vi "WHD_VEten_0.1.6.WS_BIDIR_Cal_26_01_2024.vi"() -> ()   [LabVIEW 2015]
uses:
  <vilib>/LabVIEW Targets/FPGA/cRIO/shared/nicrio_ModuleControls/nicrio_cRIO-9234_DataRatesRing2.ctl
  <vilib>/RTwatchdog.llb/Watchdog expiration actions.ctl
  <vilib>/userdefined/High Color/nirio_resource_hc.ctl
  <vilib>/Platform/TimedLoop/XDataNode/timing_clust.ctl
  <vilib>/Platform/TimedLoop/XDataNode/nitl_modes.ctl
  <vilib>/Platform/TimedLoop/XDataNode/wakeup.ctl
  <vilib>/Analysis/5stat.llb/RMS (DBL).vi
  <vilib>/FPGAPlugInAG/cRIO-9031/niLvFpga_Open_cRIO-9031.vi
  <vilib>/Utility/error.llb/Error Cluster From Error Code.vi
  <vilib>/rvi/errors/niLvFpgaAdjustHostInterfaceError.vi
  <vilib>/FPGAPlugInAG/cRIO-9031/niLvFpga_Run_cRIO-9031.vi
  <vilib>/rvi/interface/common/niFpgaWaitOnOcc.vi
  <vilib>/Utility/file.llb/Write Delimited Spreadsheet (string).vi
  <vilib>/FPGAPlugInAG/cRIO-9031/niLvFpga_Reset_cRIO-9031.vi
  <vilib>/measure/madcrms.llb/Basic Averaged DC-RMS for 1 Chan.vi
  <vilib>/measure/maspectr.llb/FFT Spectrum (Mag-Phase) for 1 Chan.vi
  <vilib>/Utility/config.llb/Write Key (Double).vi
  <vilib>/FPGAPlugInAG/cRIO-9031/niLvFpga_Close_cRIO-9031.vi
  <vilib>/rvi/interface/nirviOpenFPGA/nirviOpenFPGA.xnode
  FPGA Bitfiles/WRDArabia_FPGATarget_FPGA8a2wsBIdirec_pdg683fU6LY.lvbitx
  <vilib>/rvi/interface/nirviReadWriteControl/nirviReadWriteControl.xnode
  <vilib>/rvi/interface/nirviMethod/nirviMethod.xnode
  <vilib>/platform/TimedLoop/XDataNode/XDataNode.xnode
  <vilib>/rvi/interface/nirviCloseFPGA/nirviCloseFPGA.xnode
  <vilib>/NI_Real-Time Target Support.lvlib
  <vilib>/rvi/errors/niLvFpgaMergeErrorWithErrorCode.vi
  AURA_Wheel/Json2Labv.lvlib
  AURA_Wheel/AuraWheelAPI/AuraWheel.lvlib
  NiFpgaLv.dll
  <vilib>/FPGAPlugInAG/cRIO-9031/niLvFpga_ConfigureFifo_cRIO-9031.vi
  <vilib>/FPGAPlugInAG/cRIO-9031/niLvFpga_StartFifo_cRIO-9031.vi
  <vilib>/FPGAPlugInAG/cRIO-9031/niLvFpga_ReadFifo_cRIO-9031.vi
  <vilib>/FPGAPlugInAG/cRIO-9031/niLvFpga_StopFifo_cRIO-9031.vi
  <vilib>/measure/NI_MAPro.lvlib
  <vilib>/Analysis/NI_AALPro.lvlib
  <vilib>/Analysis/NI_AALBase.lvlib
  <vilib>/Utility/config.llb/NI_LVConfig.lvlib
  <vilib>/Platform/TimedLoop/XDataNode/XDNodeRunTimeDep.lvlib
  Library/IF2_Reader/IF2_Reader.lvlib
panel:
  out "t":string
  out "Diagnostic data":sgl[](array[numeric])
  out "Last Train passes - RFIDs":T1
  out "I2":sgl[](array[numeric])
  out "I1":sgl[](array[numeric])
  out "A8":sgl[](array[numeric])
  out "A7":sgl[](array[numeric])
  out "A6":sgl[](array[numeric])
  out "A5":sgl[](array[numeric])
  out "A4":sgl[](array[numeric])
  out "A3":sgl[](array[numeric])
  out "A2":sgl[](array[numeric])
  out "A1":sgl[](array[numeric])
  out "Accelerometer 8":bool
  out "Accelerometer 7":bool
  out "Accelerometer 6":bool
  out "Accelerometer 5":bool
  out "Accelerometer 4":bool
  out "Accelerometer 3":bool
  out "Accelerometer 2":bool
  out "Accelerometer 1":bool
  out "Wheel detector 2":bool
  out "Wheel Detector 1":bool
  out "Last time checked":string
  out "RFID connection":bool
  out "Internet connection":bool
  out "Inicio diagnosis":timestamp
  out "RFID_status":path=path "c:/RFID/status.csv"
  in  "Diagnosis":bool
  out "T fuera rango":bool
  out "Frequency":dbl[](array[numeric])
  out "Value to compare":dbl[](array[numeric])
  in  "Developer password":string
  out "Waveform Graph":waveform(sgl)[](graph)
  out "min":dbl[](array[numeric])
  out "max":dbl[](array[numeric])
  out "median":dbl[](array[numeric])
  out "mean":dbl[](array[numeric])
  in  "Accelerometer":i32=1 min=1 max=8
  out "Low cutoff freq":dbl
  out "noise_range":dbl
  out "Numeric":i32
  out "Calibration parameter":dbl
  out "Accel.detected":i32
  out "Mean\nfrequency":dbl format="%0.2f"
  out "Nº meas":i32
  out "Array":i32[](array[numeric])
  out "sorted array":i32[](array[numeric])
  out "Array 3":i32[](array[numeric])
  out "max value":i32
  out "max index(es)":i32
  out "element":i32
  out "size(s) 3":i32
  out "size(s)":i32[](array[numeric])
  out "Valid\nindex":i32[](array[numeric])
  out "Acquiring time":dbl
  out "Inicio pasada 2":timestamp
  out "calibration log":path
  out "date/time string 2":string
  out "Folder":path
  in  "Developer commad":string
  out "Save calibration":bool
  out "Pattern amplitude (g)":dbl=1.02
  out "Pattern frequency (Hz)":dbl=159.2
  out "Report":string
  out "AURA wheel test":bool
  out "LOG.txt":path
  out "Report_AURA":string
  out "error FPGA":errorcluster
  out "error AURA":errorcluster
  out "error manipulacion archivos":errorcluster
  out "Response headers":string
  out "Max RMS Ruedas":dbl[][](array[numeric])
  out "TAGs LR6":string[](array[string])
  out "TAGs HEX":string[](array[string])
  out "Parar":bool
  out "result":bool
  out "TAGs":string[](array[string])
  out "Temperatura (ºC)":dbl
  out "V (m/s)":dbl
  out "Digital?":bool=TRUE
  out "Watchdog config":T2={"reset"=FALSE, "occurrence"=FALSE, "trigger protocol"=enum."active high", "trigger line"=enum."none", "disable watchdog on VI exit"=TRUE}
  out "Tiempo de adquisicion":dbl=10.0
  out "Adquirir":bool
  out "Nº Ruedas 1":i32
  out "NºRuedas 2":i32
  out "Disco Duro Disponible (bytes)":i64
  out "Buffer Overflow":bool
  out "Buffer Underflow":bool
  out "Archivo\nvalido?":bool
  out "Número de ejes detectados":i32
  out "Ejes_convoy":i32
  out "Tiempo de paso (s)":dbl
  out "created path":path
  out "Nombre de archivo":path[](array[path])
  out "LR6 IP address":string="192.168.106.94"
  out "Port LR6":u16=2001
  out "Frecuencia de muestreo (Hz)":dbl=25600.0
  out "Escaneos de la FIFO por canal":u32=5000
  out "Tiempo extra al detector de paso (s)":dbl=1.0
  out "dt RMS":dbl=256.0
  out "Frecuencia de muestreo y módulo CRIO":T3=2 items=["51.200 kS/s (NI 9234)"=1, "25.600 kS/s (NI 9234)"=2, "17.067 kS/s (NI 9234)"=3, "12.800 kS/s (NI 9234)"=4, "10.240 kS/s (NI 9234)"=5, "8.533 kS/s (NI 9234)"=6, "7.314 kS/s (NI 9234)"=7, "6.400 kS/s (NI 9234)"=8, "5.689 kS/s (NI 9234)"=9, "5.120 kS/s (NI 9234)"=10, "4.654 kS/s (NI 9234)"=11, "4.267 kS/s (NI 9234)"=12, "3.938 kS/s (NI 9234)"=13, "3.657 kS/s (NI 9234)"=14, "3.413 kS/s (NI 9234)"=15, "3.200 kS/s (NI 9234)"=16, "3.012 kS/s (NI 9234)"=17, "2.845 kS/s (NI 9234)"=18, "2.695 kS/s (NI 9234)"=19, "2.560 kS/s (NI 9234)"=20, "2.438 kS/s (NI 9234)"=21, "2.328 kS/s (NI 9234)"=22, "2.226 kS/s (NI 9234)"=23, "2.133 kS/s (NI 9234)"=24, "2.048 kS/s (NI 9234)"=25, "1.969 kS/s (NI 9234)"=26, "1.896 kS/s (NI 9234)"=27, "1.829 kS/s (NI 9234)"=28, "1.765 kS/s (NI 9234)"=29, "1.707 kS/s (NI 9234)"=30, "1.652 kS/s (NI 9234)"=31]
  out "Puerto RFID":u16=2189
  out "IP RFID":string="192.168.106.99"
  out "Offset_rueda WS 2":fxp<+/-,24,-4>=0.004999998956918716 format="%.27g"
  out "Count(mSec)":u32=2
  out "RFID NEM on?":bool
  out "RFID LR6 on?":bool
  out "Canal cero WS1?":bool
  out "Canal cero WS2":bool
  in  "Calibration":bool
  out "Direccion 0?":bool
  out "Boton Adquirir?":bool
  out "RuedaDetectada2?":bool=TRUE
  out "RuedaDetectada1?":bool=TRUE
  out "Timeout ruedas":dbl
  out "Borrar archivos\nadquisicion con error":bool
  out "Able watchdog?":bool
  out "Reset watchdog?":bool
  out "Leer config RFID NEM":bool
  out "bytes to read":i32
  out "DeviceAddress":u8
  out "timeout ms (60000)":i32
  out "Max archivos":u32=2
  out "Bytes libre despues de borrar":u32=2
  out "Bytes min libre":u32=2
  out "Nº de acelerómetros":i32
  out "Nº inductivos":i32
  out "Offset_rueda WS 1":fxp<+/-,24,-4>=0.004999998956918716 format="%.27g"
  out "TAGs_AURAwheel":string[][](array[string])
  out "Plataformas?":bool
  out "Nº Ejes":i32[](array[numeric])
  out "Nº UTs":i32
  out "it-read-LR6":i32[](array[numeric])
  out "it-LR6":i32
  out "RFID_LR6_Error":errorcluster
  out "Series_flota":string[](array[string])
  out "Tabla_flota":string[][](array[string])
  out "Puntos medios de las ventanas":dbl[][](array[numeric])
  out "configuration file path":path=path "c:/Parametros.cfg"
  out "IP synchr":string
  out "data":cluster{"status":string}
  out "confRFID":path=path "c:/RFID/TAGS.csv"
  out "TAGS leidos":path=path "c:/RFID/TAGS.csv"
  out "Use Aura?":bool
  out "Parametros AuraWheel":string[](array[string])
  out "Parámetros acelerómetros":dbl[](array[numeric])
  out "Fin":bool
  out "Contador":i32=1
  out "Path LOG":path=path "c:/TEST"
  out "Fallo fotocelula":bool
  out "Path_Borrar":path=path "c:/Trenes"
  out "Longitud de la unidad":dbl
  out "Aviso no detección":string
  out "Time to Acquire Block (ms)":i32
  out "Distancia de acelerómetros":dbl[](array[numeric])
  out "Block Size":u32
  out "Distancias generales":dbl[](array[numeric])
  out "Reset del controlador":bool
  out "Parar la aplicación":bool
  out "date/time string":string
  out "Timeout ruedas":bool
  out "Tiempo":dbl
  out "Inicio pasada":timestamp
  out "Ultimo TEST":timestamp
  out "Fuente":bool=TRUE
  out "DC OK":string
  out "Aviso temperatura":string
  out "connection ID":refnum<k5>
  # "To check the status of the UPS please check the following LEDs physically in the system:"
  # "10. Bar graph showing the current available supply of the UPS (each bar is a 20%)"
  # "12. Red LED: alarm"
  # "13. Yellow LED: battery working mode"
  # "16. Green LED: Power In OK, mains mode"
  # "Calibration - Noise analysis"
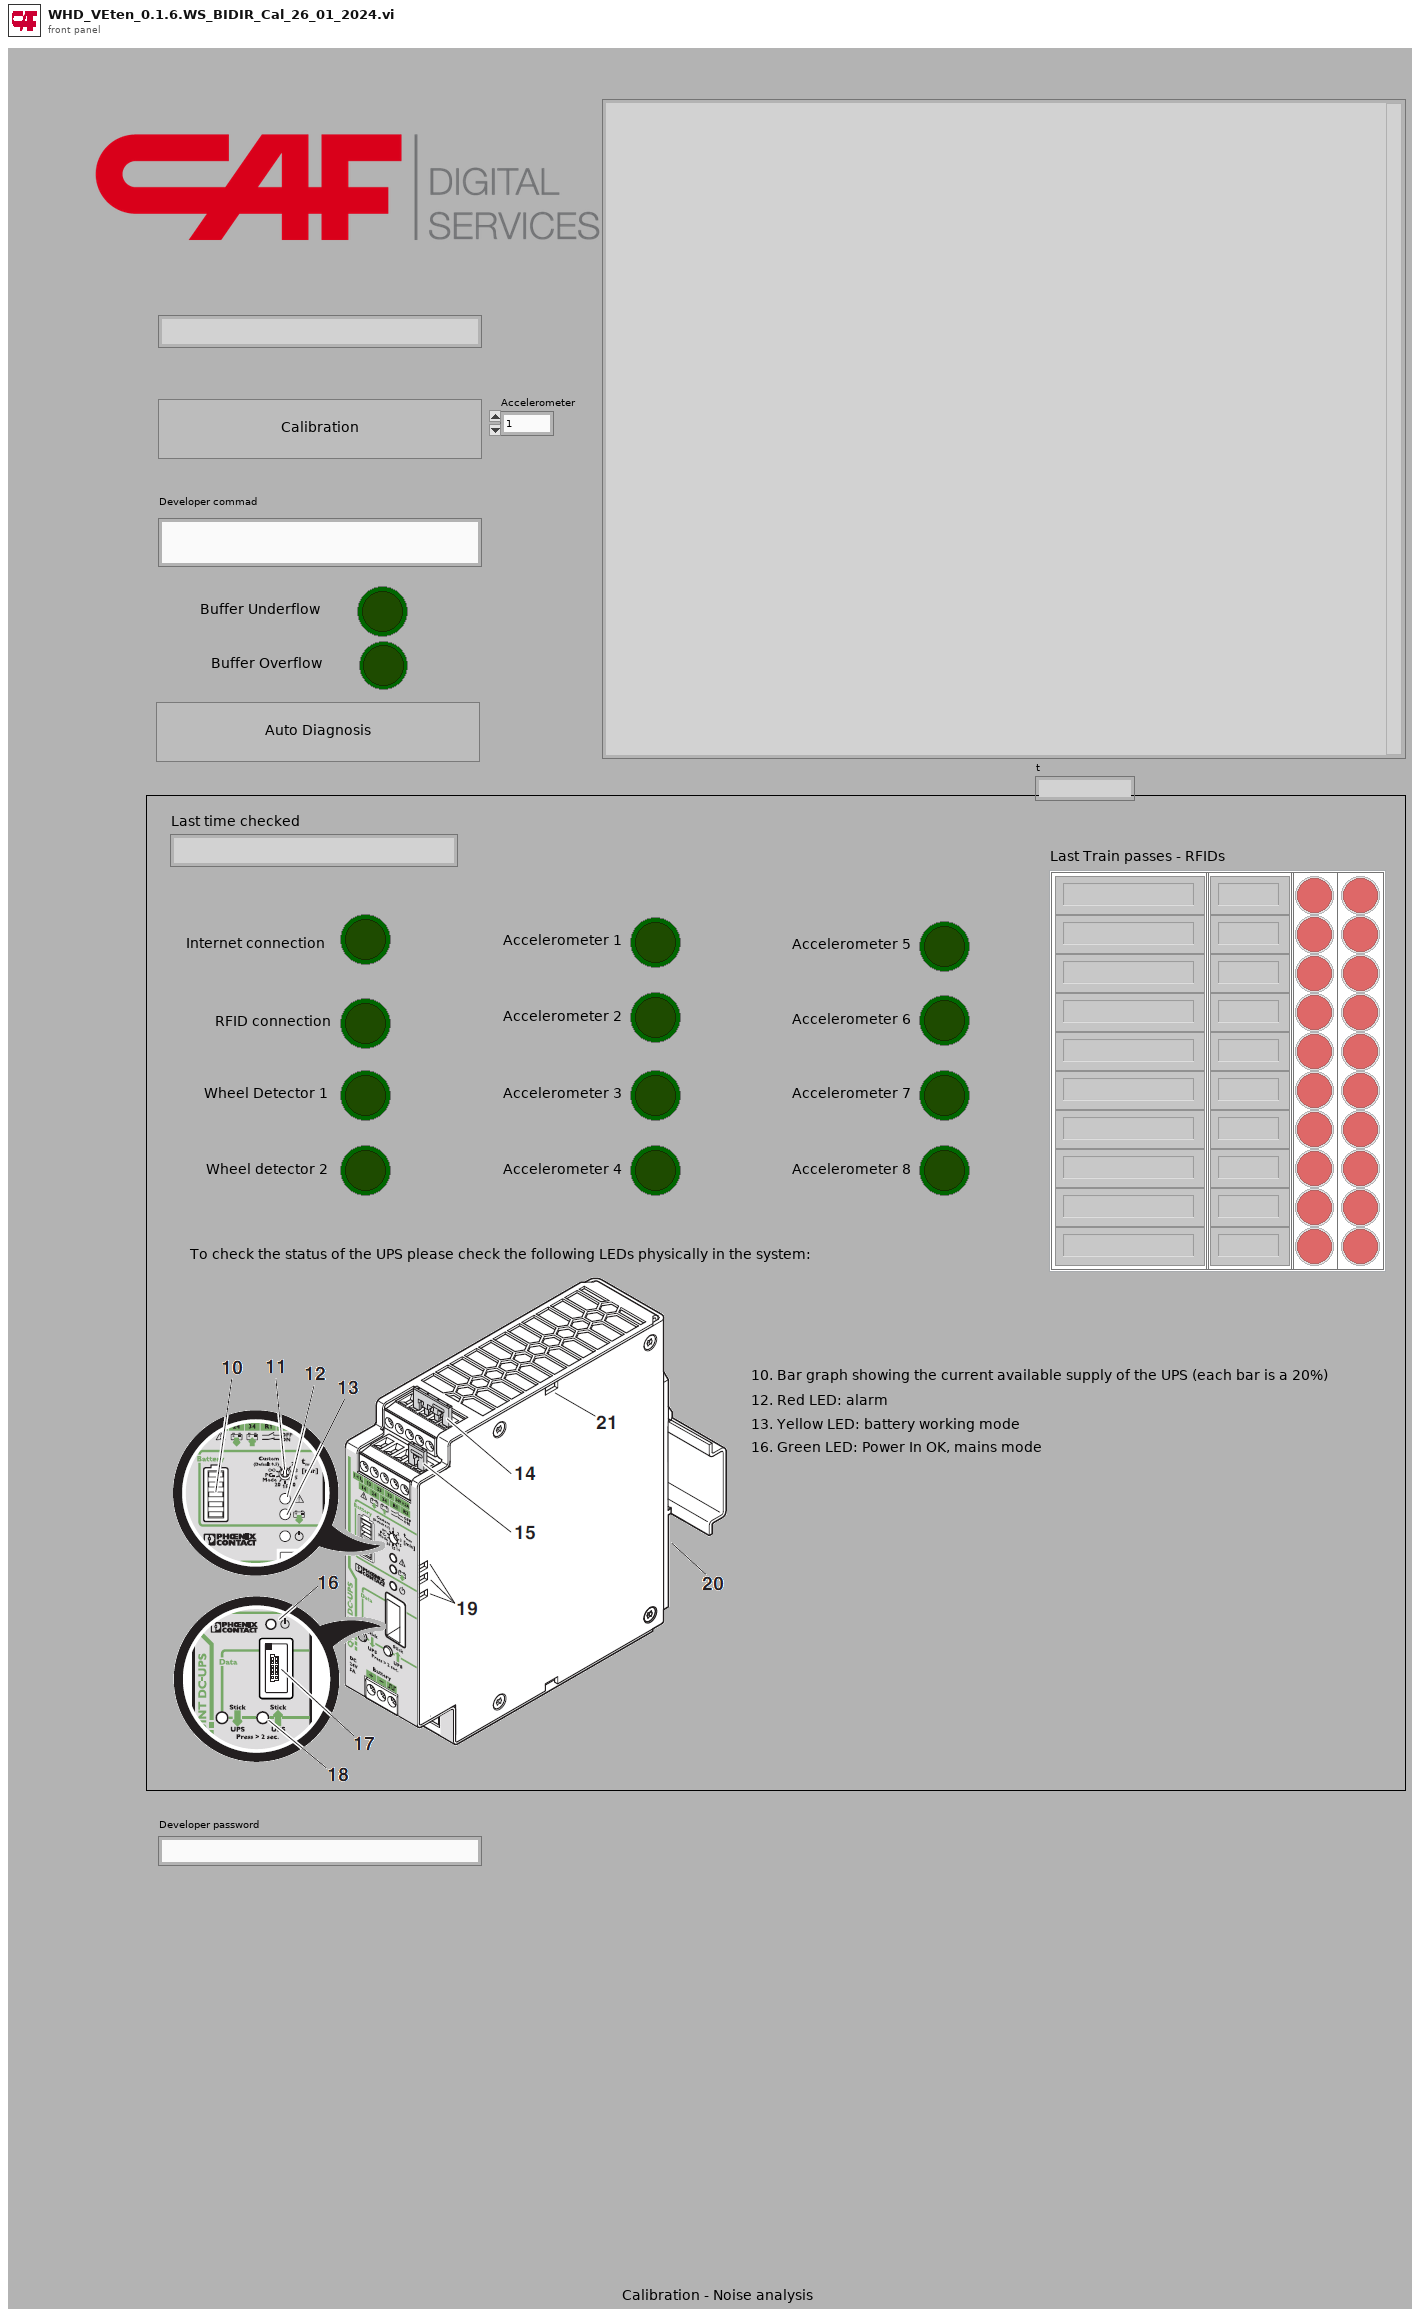
[diagram p1: front panel]
types:
  T1 = cluster{"Array 3":bool[], "Array 4":string[], "Array 6":string[], "Array 5":bool[]}
  T2 = typedef "Watchdog expiration actions.ctl" = cluster{"reset":bool, "occurrence":bool, "trigger protocol":enum16{"active high", "active low", "open collector"}, "trigger line":enum16{"none", "line 0", "line 1", "line 2", "line 3", "line 4", "line 5", "line 6", "line 7", "SMB line 0"}, "disable watchdog on VI exit":bool}
  T3 = typedef "nicrio_cRIO-9234_DataRatesRing2.ctl" = u8
  T4 = typedef "nirio_resource_hc.ctl" = tag
  T5 = enum16{"open", "replace", "create", "open or create", "replace or create", "replace or create with confirmation"}
  T6 = enum16{"big-endian, network order", "native, host order", "little-endian"}
  T7 = typedef "XDNodeRunTimeDep.lvlib/timing_clust.ctl" = cluster{"Expected End [f-1]":u64, "Actual End [f-1]":u64, "Finished Late? [f-1]":bool, "Expected End [i-1]":u64, "Actual End [i-1]":u64, "Finished Late? [i-1]":bool, "Expected Start [i]":u64, "Actual Start [i]":u64, "Expected Start [f]":u64, "Actual Start [f]":u64, "Source Name":string, "Structure Name":string, "Period":i64, "Deadline":i64, "Offset":i64, "Start":i64, "Priority":i32, "Timeout":i32, "Mode":T8, "Wakeup Reason":T9, "Error":errorcluster, "Source Type":string, "Secondary Source Type":string, "Global End Time":u64, "Global Start Time":u64, "Frame Duration":u64, "Iteration Duration":u64, "Assigned CPU":i32, "I/O Scan Engine Mode":u32}
  T8 = typedef "XDNodeRunTimeDep.lvlib/nitl_modes.ctl" = enum32{"No Change", "Process missed periods, maintain original phase", "Discard missed periods, maintain original phase", "Process missed periods, ignore original phase", "Discard missed periods, ignore original phase"}
  T9 = typedef "XDNodeRunTimeDep.lvlib/wakeup.ctl" = enum32{"Normal", "Aborted", "Asynchronous wakeup", "Timing source error", "Timed loop error", "Timeout"}
  T10 = cluster{"error IO":errorcluster, bool[], u32[], string[], dbl[]}
  T11 = cluster{"error out":errorcluster, dbl[], "Normalized Tags":string[], "Direccion 0?":bool}
  T12 = cluster{"g_ts":dbl, "p_sp":dbl, "p_tp":dbl, "p_tg":cluster{"tg_n":dbl, "tg_t":string}[], "p_ax":cluster{"ax_n":dbl, "ax_sp":dbl, "ax_wh":cluster{"wh_p":dbl, "wh_a1":dbl, "wh_a2":dbl, "wh_a3":dbl, "wh_a4":dbl}[]}[]}
  T13 = typedef "NI_LVConfig.lvlib/Config Data RefNum.ctl" = refnum<k1>
  T14 = cluster{"IP":string, "Port":u16, "ReaderConfigFile":path, "ROspecConfigFile":path}
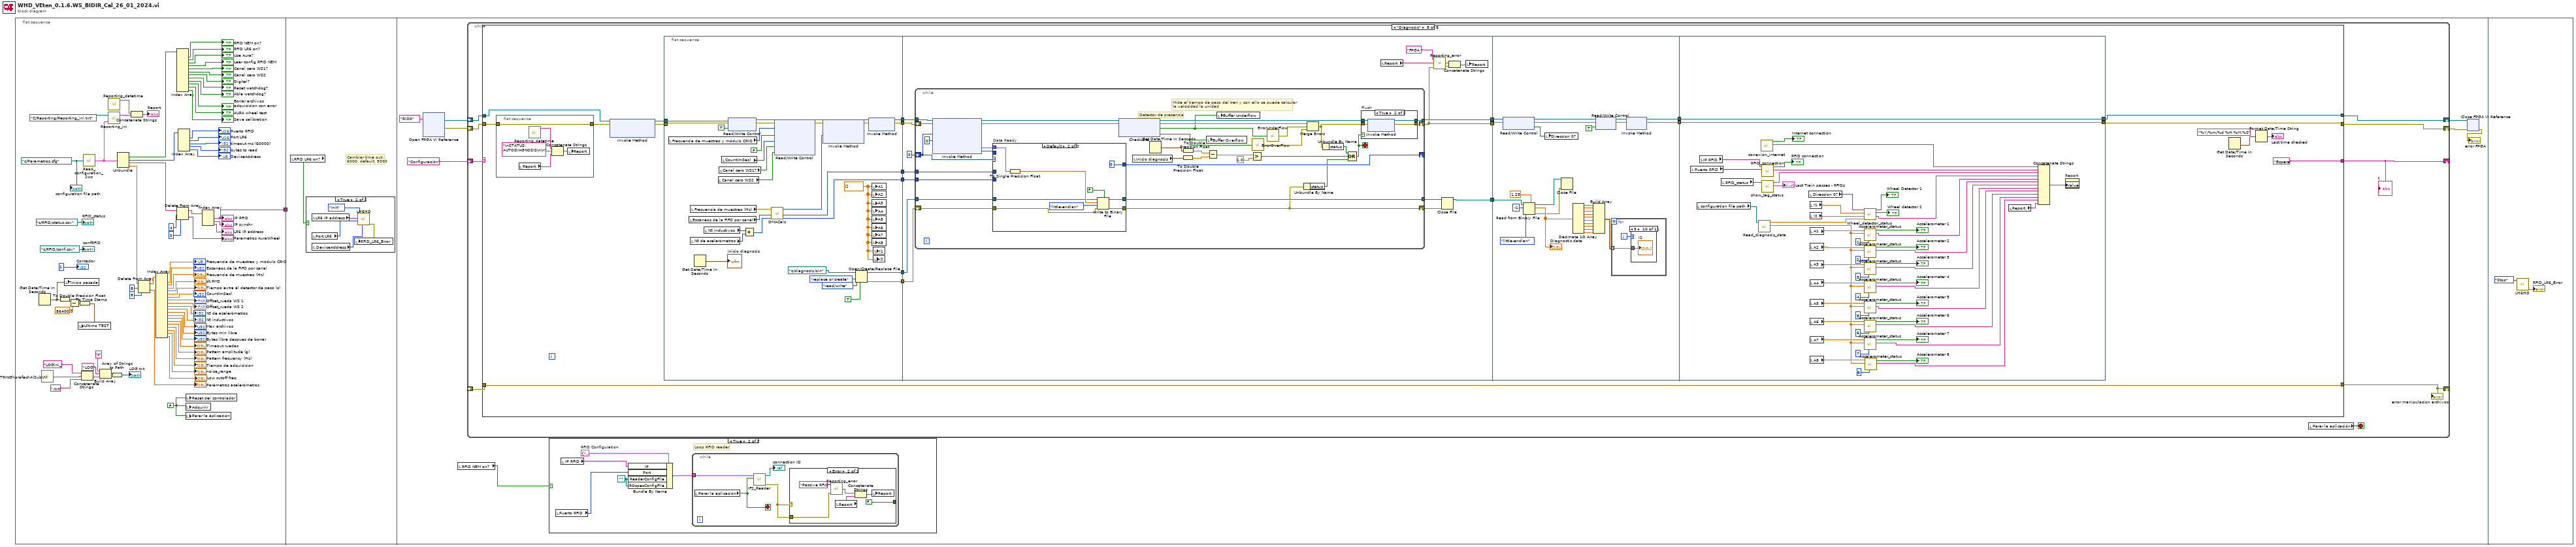
[diagram p0: block diagram]
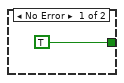
[diagram p4: hidden frame]
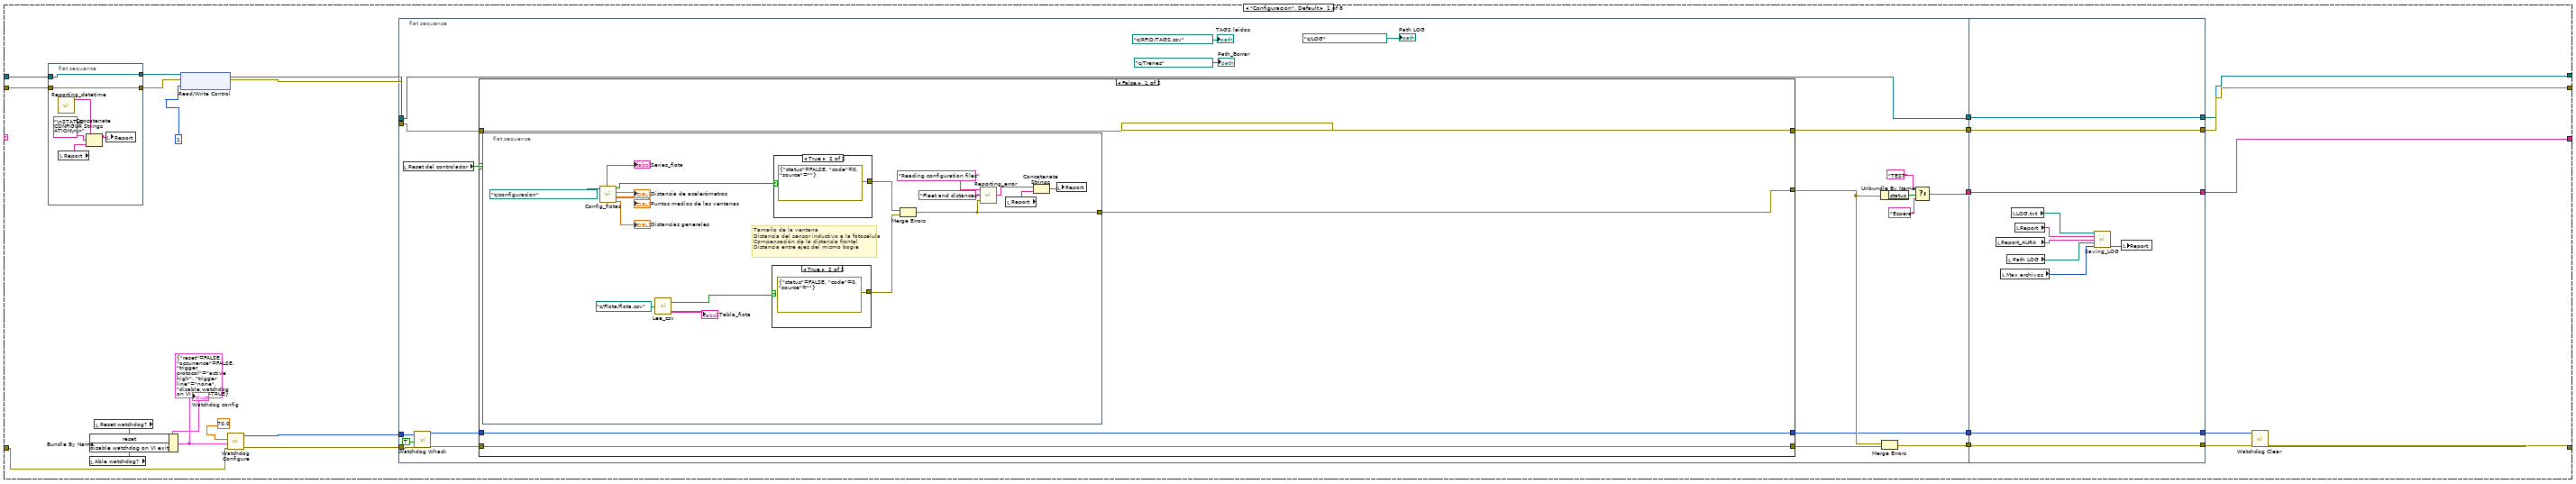
[diagram p5: hidden frame]
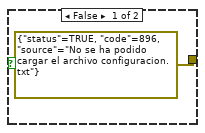
[diagram p6: hidden frame]
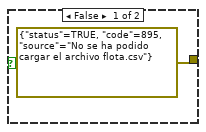
[diagram p7: hidden frame]
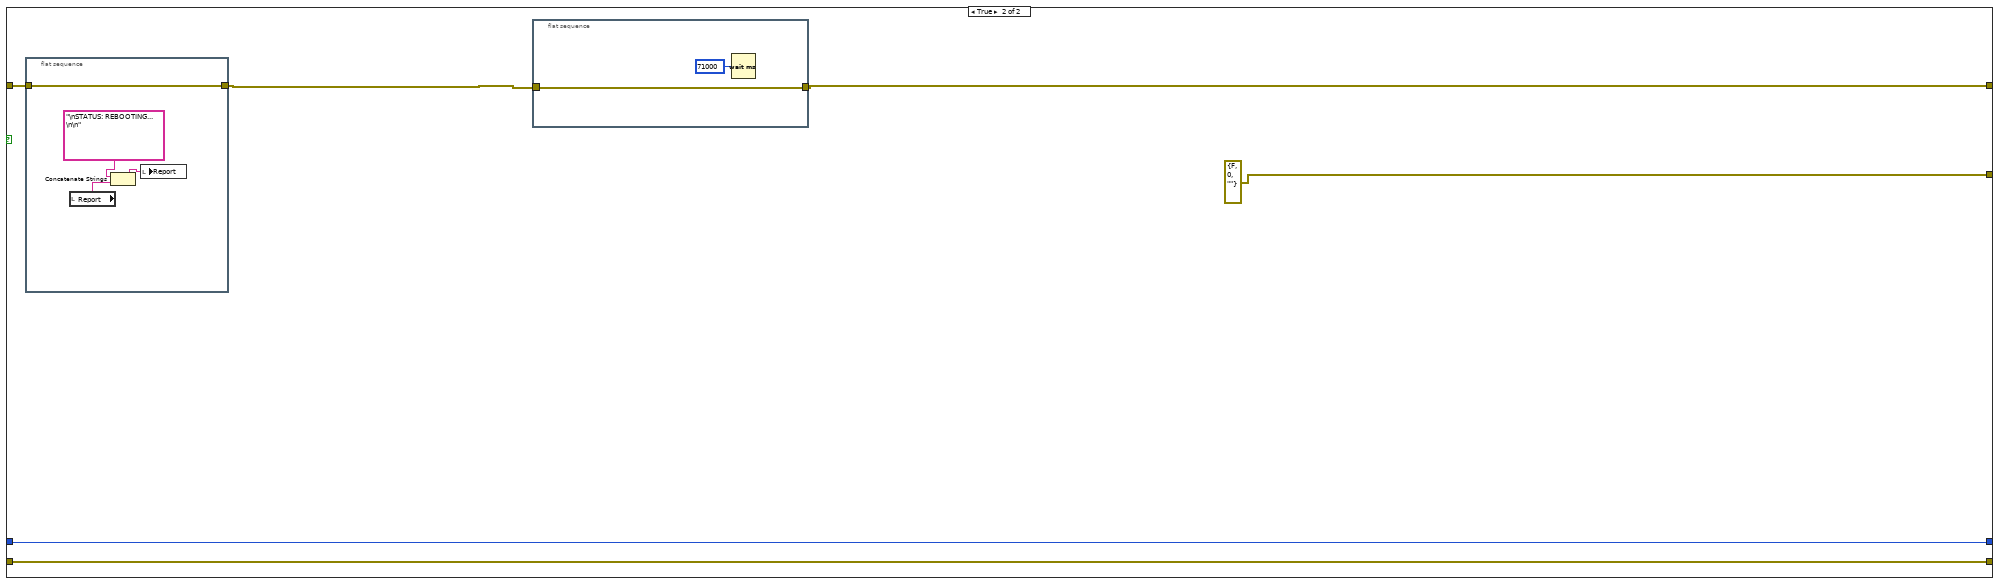
[diagram p8: hidden frame]
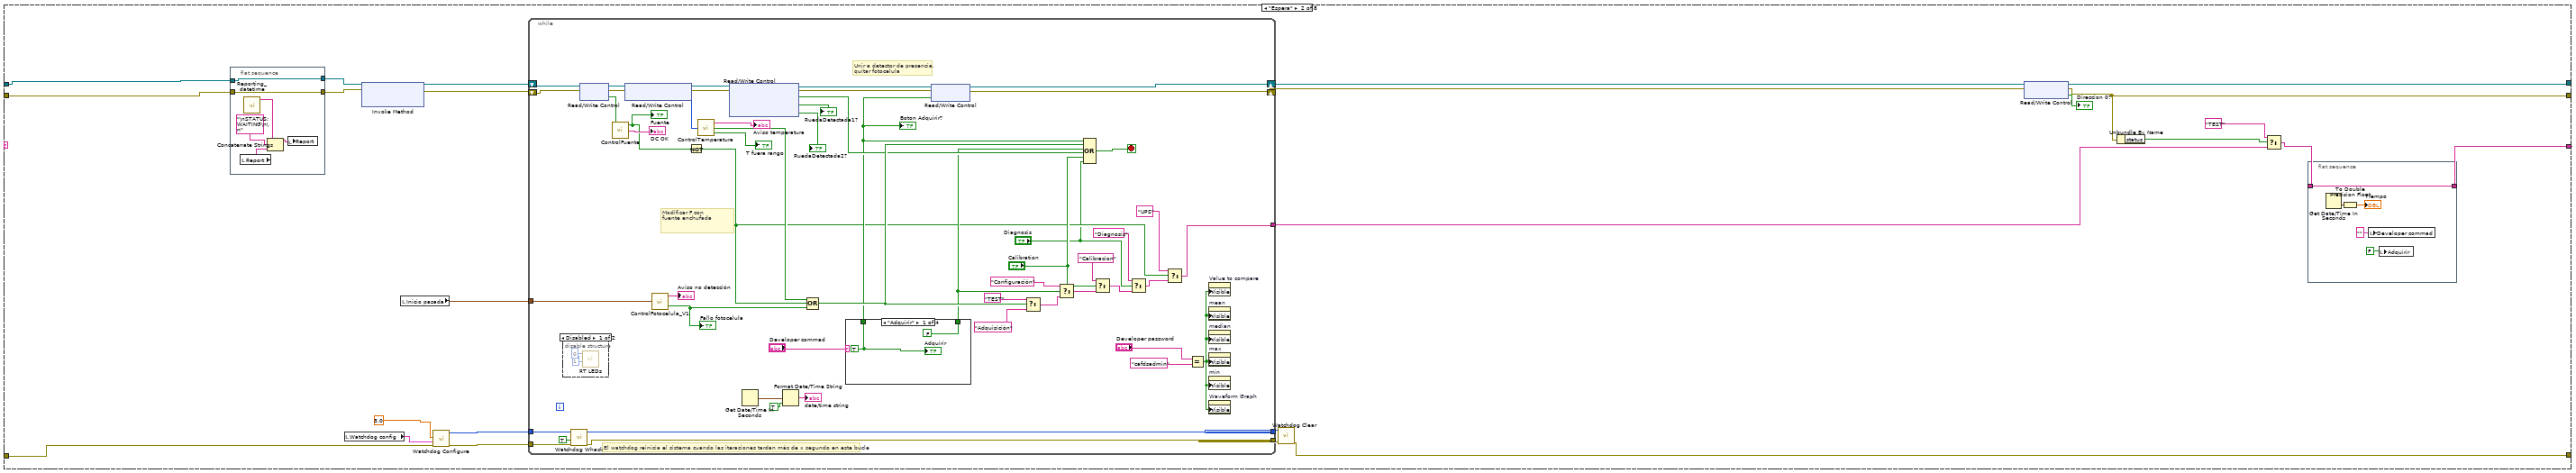
[diagram p9: hidden frame]
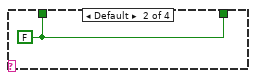
[diagram p10: hidden frame]
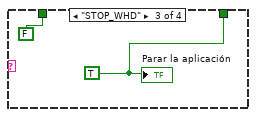
[diagram p11: hidden frame]
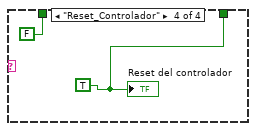
[diagram p12: hidden frame]
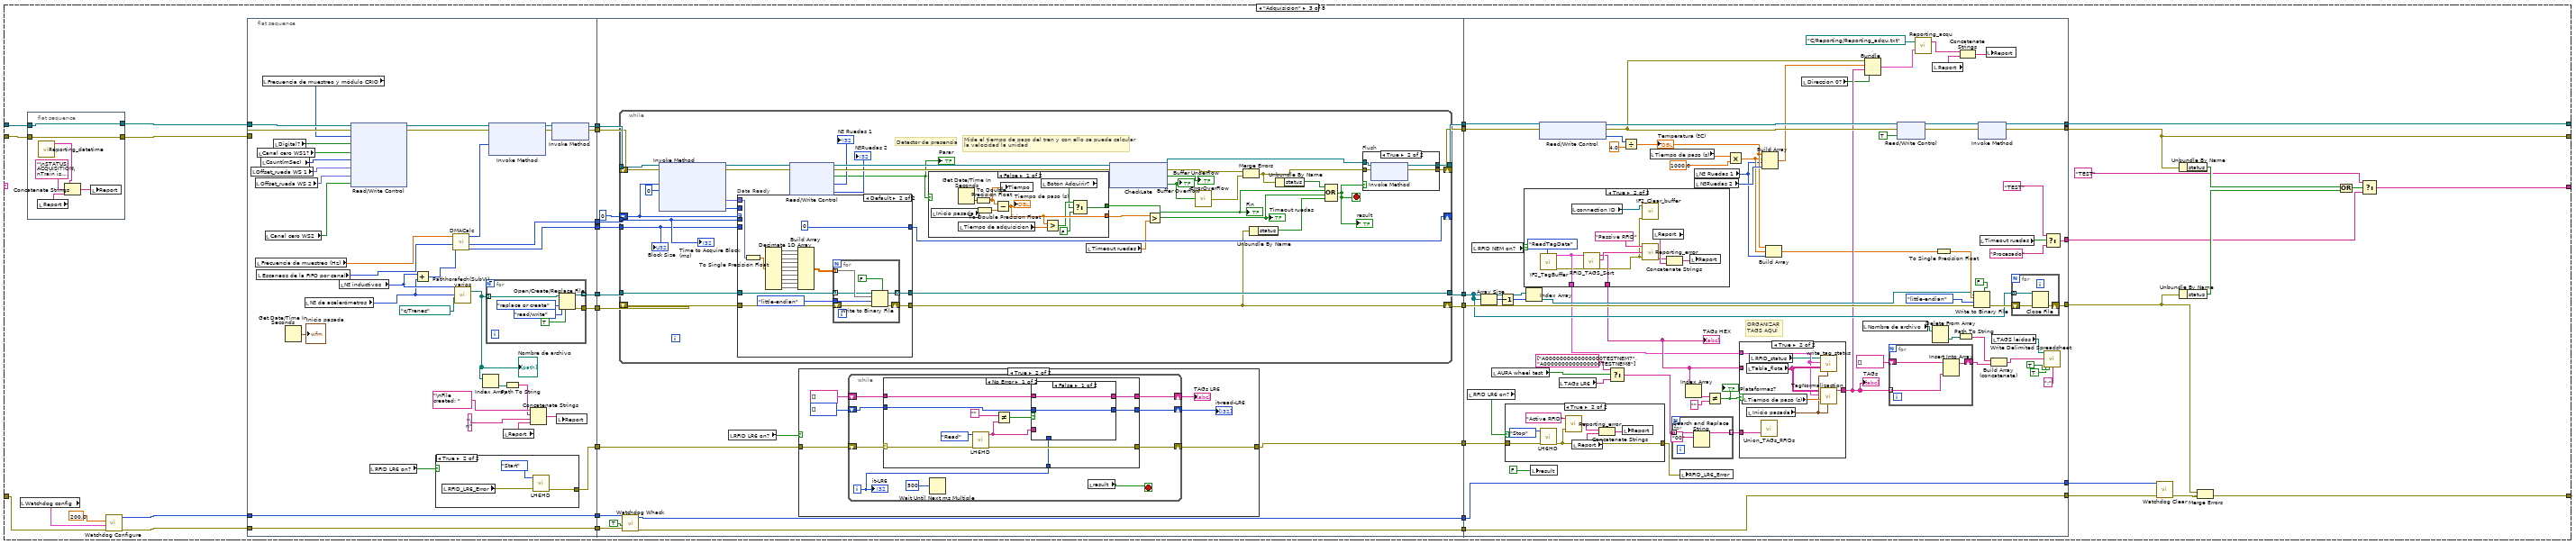
[diagram p14: hidden frame]
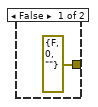
[diagram p15: hidden frame]
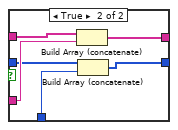
[diagram p17: hidden frame]
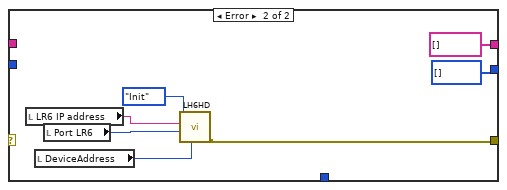
[diagram p18: hidden frame]
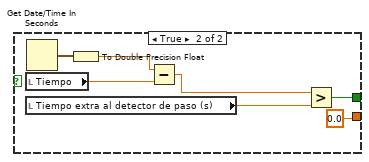
[diagram p19: hidden frame]
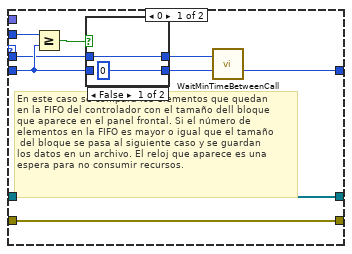
[diagram p20: hidden frame]
diagram:
  n1 = flat-sequence {
    tunnel: [w5] -> w1
    tunnel: w1 -> [_]
    frame #0 {
      w6 = FALSE ("Reset del controlador")
      w67 = path "c:/Parametros.cfg" ("configuration file path")
      n2 = Get Date/Time In Seconds() -> (seconds since 1Jan1904=w72:timestamp)
      n3 = call "STRINGhorafechA(SubVI).vi"() -> ("STRINGhora_fecha"=w17:string)
      n4 = To Double Precision Float(number=w72) -> (double precision float=w74:dbl)
      n5 = local write "Inicio pasada"(w72) -> ()
      n6 = Subtract(x=w74, y=86400.0) -> (x-y=w73:dbl)
      n7 = To Time Stamp(1:w73) -> (0:w71:timestamp)
      n8 = local write "Ultimo TEST"(w71) -> ()
      n9 = Concatenate Strings("LOGini_" ("string"), w17, ".txt" ("string")) -> (w19:string)
      n10 = call "Read_configuration_2ws.vi"("configuration file path"=w67) -> ("output cluster"=w23:T10)
      n11 = Build Array("c", "LOG" ("element"), w19) -> (w16:string[])
      n12 = call "Reporting_ini.vi"("Configuration cluster"=w23, "address repoting"=path "C:/Reporting/Reporting_ini.txt" ("file (use dialog)")) -> ("Reporting"=w22:string)  [unwired: 1 in]
      n13 = call "Reporting_datetime.vi"() -> ("String"=w20:string)  [unwired: 11 in]
      n14 = Array of Strings to Path(0:w16) -> (2:→"LOG.txt":path)  [unwired: 1 out]
      n15 = Unbundle(w23) -> (w70:bool[], w69:u32[], w62:string[], w66:dbl[])  [unwired: 1 out]
      n16 = Concatenate Strings(w20, w22) -> (→"Report":string)
      n17 = Delete From Array(array=w66, length=8, index=8) -> (deleted portion=→"Parámetros acelerómetros":dbl[], array with subset deleted=w65:dbl[])
      n18 = Index Array(array=w65) -> (element #1=→"Frecuencia de muestreo y módulo CRIO":dbl, element #2=→"Escaneos de la FIFO por canal":dbl, element #3=→"Frecuencia de muestreo (Hz)":dbl, element #4=→"dt RMS":dbl, element #5=→"Tiempo extra al detector de paso (s)":dbl, element #6=→"Count(mSec)":dbl, element #7=→"Offset_rueda WS 1":dbl, element #8=→"Offset_rueda WS 2":dbl, element #9=→"Nº de acelerómetros":dbl, element #10=→"Nº inductivos":dbl, element #11=→"Max archivos":dbl, element #12=→"Bytes min libre":dbl, element #13=→"Bytes libre despues de borrar":dbl, element #14=→"Timeout ruedas":dbl, element #15=→"Pattern amplitude (g)":dbl, element #16=→"Pattern frequency (Hz)":dbl, element #17=→"Tiempo de adquisicion":dbl, element #18=→"noise_range":dbl, element #19=→"Low cutoff freq":dbl)  [unwired: 19 in]
      n19 = Index Array(array=w70) -> (element #1=→"RFID NEM on?":bool, element #2=→"RFID LR6 on?":bool, element #3=→"Use Aura?":bool, element #4=→"Leer config RFID NEM":bool, element #5=→"Canal cero WS1?":bool, element #6=→"Canal cero WS2":bool, element #7=→"Digital?":bool, element #8=→"Reset watchdog?":bool, element #9=→"Able watchdog?":bool, element #10=→"Borrar archivos\nadquisicion con error":bool, element #11=→"AURA wheel test":bool, element #12=→"Save calibration":bool)  [unwired: 12 in]
      n20 = Delete From Array(array=w62, length=4, index=0) -> (deleted portion=→"Parametros AuraWheel":string[], array with subset deleted=w61:string[])
      n21 = Index Array(array=w69) -> (element #1=→"Puerto RFID":u32, element #2=→"Port LR6":u32, element #3=→"timeout ms (60000)":u32, element #4=→"bytes to read":u32, element #5=→"DeviceAddress":u32)  [unwired: 5 in]
      n22 = local write "Reset del controlador"(w6) -> ()
      n23 = local write "Adquirir"(w6) -> ()
      n24 = local write "Parar la aplicación"(w6) -> ()
      n25 = Index Array(array=w61) -> (element #1=w5:string, element #2=→"IP synchr":string, element #3=→"LR6 IP address":string)  [unwired: 3 in]
      "IP RFID" <- w5
      "Contador" <- 1
      "confRFID" <- path "c:/RFID/conf.csv" ("file path (use dialog)")
      "configuration file path" <- w67
      "RFID_status" <- path "c:/RFID/status.csv" ("file path (use dialog)")
    }
    frame #1 {
      # "Cambiar time out:\n6000, default, 5000"
      n26 = local read "RFID LR6 on?"() -> (w76:bool)
      n27 = case shown="True" w76 {
        frame False {
        }
        frame True {
          n28 = local read "LR6 IP address"() -> (w77:string)
          n29 = local read "Port LR6"() -> (w78:u16)
          n30 = local read "DeviceAddress"() -> (w79:u8)
          n31 = call "LH6HD.vi"("DeviceAddress"=w79, "Reader Port"=w78, "IP Address"=w77, "Action"=enum16{"Init", "Start", "Read", "Stop", "Exit"}."Init") -> ("error out"=w81:errorcluster)  [unwired: 6 in, 1 out]
          n32 = local write "RFID_LR6_Error"(w81) -> ()
        }
      }
    }
    frame #2 {
      n33 = xnode "Open FPGA VI Reference"("resource name"=T4 "RIO0") -> ("FPGA VI Reference Out"=w89:refnum<k20>, "error out"=w88:errorcluster)  [unwired: 1 in]
      n34 = local read "RFID NEM on?"() -> (w82:bool)
      n35 = while {
        shift-right: [w107] -> _
        shift-left: "Configuración" -> [w114]
        shift-right: [w106] -> w85
        shift-left: w89 -> [w113]
        shift-right: [w108] -> w84
        shift-left: w88 -> [w112]
        shift-right: [w111] -> _
        shift-left: _ -> [w110]
        stop <- w109 stop-if-true
        n36 = case shown="\"Diagnosis\"" w114 {
          tunnel: [w129 w232 w330 w681 w929 "Espera" "Espera" ("t") "Espera" ("t")] -> w107
          tunnel: [w139 w221 w344 w670 w928 w997 w1798 w1820] -> w106
          tunnel: [w140 w220 w345 w668 w927 w995 w1797 w1829] -> w108
          tunnel: w113 -> [w123 w219 w316 w671 w928 w1007 w1799 w1838]
          tunnel: w112 -> [w122 w218 w315 w669 w920 w1006 w1794 w1840]
          tunnel: [w136 w226 w342 w666 w919 w996 w1795 w1821] -> w111
          tunnel: w110 -> [w128 w231 w326 w680 w916 w996 w1795 w1821]
          frame "Configuración", Default {
            n37 = flat-sequence {
              tunnel: w123 -> [w146]
              tunnel: w122 -> [w145]
              tunnel: [w146] -> w121
              tunnel: [w145] -> w120
              frame #0 {
                n38 = call "Reporting_datetime.vi"() -> ("String"=w141:string)  [unwired: 11 in]
                n39 = local read "Report"() -> (w142:string)
                n40 = Concatenate Strings(w141, "\nSTATUS: CONFIGURATION\n\n", w142) -> (w144:string)
                n41 = local write "Report"(w144) -> ()
              }
            }
            n42 = local read "Able watchdog?"() -> (w133:bool)
            n43 = local read "Reset watchdog?"() -> (w134:bool)
            n44 = Bundle By Name(cluster=T2 {"reset"=FALSE, "occurrence"=FALSE, "trigger protocol"=enum."active high", "trigger line"=enum."none", "disable watchdog on VI exit"=TRUE} ("expiration actions"), "reset"=w134, "disable watchdog on VI exit"=w133) -> (w127:T2)
            "Watchdog config" <- w127
            n45 = xnode "Read/Write Control"("FPGA VI Reference In"=w121, "error in"=w120, "Cycles to Filter"=u16 1) -> ("FPGA VI Reference Out"=w132:refnum<k20>, "error out"=w131:errorcluster)
            n46 = call <vilib>:"Watchdog Configure.vi"("error in (no error)"=w128, "expiration actions"=w127, "timeout (1 sec)"=70.0) -> ("error out"=w124:errorcluster, "watchdogID"=w125:u64)  [unwired: 1 in, 2 out]
            n47 = flat-sequence {
              tunnel: w132 -> [w158]
              tunnel: w131 -> [w155]
              tunnel: w125 -> [w148]
              tunnel: w124 -> [w147]
              tunnel: [w157] -> w119
              tunnel: [w165] -> w118
              tunnel: [w158] -> w117
              tunnel: [w160] -> w116
              tunnel: [w152] -> w115
              tunnel: [w210] -> w138
              tunnel: [w211] -> w137
              tunnel: [w212] -> w139
              tunnel: [w213] -> w129
              tunnel: [w214] -> w140
              tunnel: w119 -> [w214]
              tunnel: w118 -> [w213]
              tunnel: w117 -> [w212]
              tunnel: w116 -> [w211]
              tunnel: w115 -> [w210]
              frame #0 {
                n48 = local read "Reset del controlador"() -> (w154:bool)
                n49 = call <vilib>:"Watchdog Whack.vi"("error in (no error)"=w147, "reset watchdog after expire? (F)"=TRUE, "watchdogID in"=w148) -> ("error out"=w150:errorcluster, "watchdogID out"=w151:u64)  [unwired: 2 in, 1 out]
                n50 = case shown="False" w154 {
                  tunnel: w155 -> [w170 w193]
                  tunnel: [w170 w196] -> w157
                  tunnel: [w167 errorcluster {"status"=FALSE, "code"=0, "source"=""} ("error IO")] -> w156
                  tunnel: [w169 w195] -> w152
                  tunnel: w151 -> [w169 w195]
                  tunnel: w150 -> [w168 w194]
                  tunnel: [w168 w194] -> w149
                  frame False {
                    n51 = flat-sequence {
                      tunnel: [w171] -> w167
                      frame #0 {
                        # "Tamaño de la ventana\nDistancia del sensor inductivo a la fotocélula\nCompensación de la distancia frontal\nDistancia entre ejes del mismo bogie"
                        n52 = call "Config_flotas.vi"("file path (dialog if empty)"=path "c:/configuracion") -> ("Distancias generales"=→"Distancias generales":dbl[], "Puntos medios de las ventanas"=→"Puntos medios de las ventanas":dbl[][], "Distancia de acelerómetros"=→"Distancia de acelerómetros":dbl[], "Distacias y medidas de dispositivos"=w184:bool, "Series_flota"=→"Series_flota":string[])  [unwired: 3 in]
                        n53 = call "Lee_csv.vi"("Path"=path "c:/Flota/flota.csv") -> ("Tabla_flota"=→"Tabla_flota":string[][], "Lectura_OK?"=w181:bool)
                        n54 = case shown="True" w181 {
                          tunnel: [errorcluster {"status"=TRUE, "code"=895, "source"="No se ha podido cargar el archivo flota.csv"} ("error out") errorcluster {"status"=FALSE, "code"=0, "source"=""} ("error out")] -> w185
                          frame False {
                          }
                          frame True {
                          }
                        }
                        n55 = case shown="True" w184 {
                          tunnel: [errorcluster {"status"=TRUE, "code"=896, "source"="No se ha podido cargar el archivo configuracion.txt"} ("error out") errorcluster {"status"=FALSE, "code"=0, "source"=""} ("error out")] -> w186
                          frame False {
                          }
                          frame True {
                          }
                        }
                        n56 = Merge Errors(w186, w185) -> (w171:errorcluster)
                        n57 = call "Reporting_error.vi"("error out 2"=w171, "Concept explanation"="Fleet and distances", "Concept"="Reading configuration files") -> ("Reporting"=w173:string)
                        n58 = local read "Report"() -> (w172:string)
                        n59 = Concatenate Strings(w173, w172) -> (w174:string)
                        n60 = local write "Report"(w174) -> ()
                      }
                    }
                  }
                  frame True {
                    n61 = flat-sequence {
                      tunnel: w193 -> [w201]
                      tunnel: [w201] -> w192
                      frame #0 {
                        n62 = local read "Report"() -> (w200:string)
                        n63 = Concatenate Strings("\nSTATUS: REBOOTING...\n\n", w200) -> (w198:string)
                        n64 = local write "Report"(w198) -> ()
                      }
                    }
                    n65 = flat-sequence {
                      tunnel: [w203] -> w196
                      tunnel: w192 -> [w203]
                      frame #0 {
                        n66 = Wait (ms)(milliseconds to wait=u32 71000) -> ()  [unwired: 1 out]
                      }
                    }
                  }
                }
                n67 = Unbundle By Name(w156) -> ("status"=w166:bool)
                n68 = Merge Errors(w156, w149) -> (w160:errorcluster)
                n69 = Select(t="TEST", s=w166, f="Espera") -> (s? t:f=w165:string)
                "Path_Borrar" <- path "c:/Trenes" ("file path (use dialog)")
                "Path LOG" <- path "c:/LOG" ("file path (use dialog)")
                "TAGS leidos" <- path "c:/RFID/TAGS.csv" ("file path (use dialog)")
              }
              frame #1 {
                n70 = local read "Report_AURA"() -> (w207:string)
                n71 = local read "Max archivos"() -> (w208:u32)
                n72 = local read "Path LOG"() -> (w209:path)
                n73 = local read "LOG.txt"() -> (w204:path)
                n74 = local read "Report"() -> (w206:string)
                n75 = call "Saving_LOG.vi"("Path"=w204, "Report"=w206, "Report AURA"=w207, "Path Carpeta"=w209, "Nº Archivos Max"=w208) -> ("Report"=w205:string)  [unwired: 9 in, 1 out]
                n76 = local write "Report"(w205) -> ()
              }
            }
            n77 = call <vilib>:"Watchdog Clear.vi"("error in (no error)"=w137, "watchdogID in"=w138) -> ("error out"=w136:errorcluster)  [unwired: 5 in]
          }
          frame "Espera" {
            n78 = flat-sequence {
              tunnel: w219 -> [w245]
              tunnel: w218 -> [w244]
              tunnel: [w245] -> w217
              tunnel: [w244] -> w216
              frame #0 {
                n79 = local read "Report"() -> (w241:string)
                n80 = call "Reporting_datetime.vi"() -> ("String"=w240:string)  [unwired: 11 in]
                n81 = Concatenate Strings(w240, "\nSTATUS: WAITING\n\n", w241) -> (w243:string)
                n82 = local write "Report"(w243) -> ()
              }
            }
            n83 = local read "Watchdog config"() -> (w225:T2)
            n84 = xnode "Invoke Method"("FPGA VI Reference In"=w217, "error in"=w216) -> ("FPGA VI Reference Out"=w235:refnum<k20>, "error out"=w234:errorcluster)  [unwired: 1 in]
            n85 = local read "Inicio pasada"() -> (w239:timestamp)
            n86 = call <vilib>:"Watchdog Configure.vi"("error in (no error)"=w231, "expiration actions"=w225, "timeout (1 sec)"=3.0) -> ("error out"=w230:errorcluster, "watchdogID"=w229:u64)  [unwired: 1 in, 2 out]
            n87 = while {
              tunnel: [w260] -> w238
              shift-right: [w275] -> w222
              shift-left: w235 -> [w283]
              shift-right: [w274] -> w215
              shift-left: w234 -> [w282]
              tunnel: w239 -> [w286]
              tunnel: w230 -> [w272]
              tunnel: w229 -> [w273]
              tunnel: [w271] -> w228
              tunnel: [w270] -> w227
              stop <- w265 stop-if-true
              # "Modificar F con\nfuente enchufada"
              # "Unir a detector de presencia,\nquitar fotocelula"
              # "El watchdog reinicia el sistema cuando las iteraciones tardan más de x segundo en este bucle"
              n88 = disable-structure shown="Disabled" {
                frame Disabled {
                  n89 = call <vilib>:"RT LEDs.vi"("State"=1, "LED Num"=0) -> ()  [unwired: 1 in, 5 out]
                }
                frame Enabled {
                }
              }
              n90 = call <vilib>:"Watchdog Whack.vi"("error in (no error)"=w272, "reset watchdog after expire? (F)"=TRUE, "watchdogID in"=w273) -> ("error out"=w270:errorcluster, "watchdogID out"=w271:u64)  [unwired: 2 in, 1 out]
              n91 = xnode "Read/Write Control"("FPGA VI Reference In"=w283, "error in"=w282) -> ("FPGA VI Reference Out"=w295:refnum<k20>, "error out"=w294:errorcluster, "DC OK"=w299:bool)
              n92 = call "ControlFuente.vi"("DC OK 3"=w299) -> ("DC OK 2"=w261:bool, "DC OK"=→"DC OK":string)  [unwired: 1 out]
              "Fuente" <- w261
              n93 = xnode "Read/Write Control"("FPGA VI Reference In"=w295, "error in"=w294) -> ("FPGA VI Reference Out"=w290:refnum<k20>, "error out"=w289:errorcluster, "Chassis Temperature"=w297:i16)
              n94 = call "ControlFotocelula_V1.vi"("Tiempo de entrada a espera"=w286) -> ("Aviso no detección"=→"Aviso no detección":string, "Boolean"=w287:bool)
              "Fallo fotocelula" <- w287
              n95 = Not(x=w261) -> (.not. x?=w259:bool)
              n96 = call "ControlTemperatura.vi"("Chassis Temperature"=w297) -> ("Aviso temperatura"=→"Aviso temperatura":string, "Boolean"=w291:bool, "T fuera rango"=→"T fuera rango":bool)
              n97 = xnode "Read/Write Control"("FPGA VI Reference In"=w290, "error in"=w289) -> ("FPGA VI Reference Out"=w285:refnum<k20>, "error out"=w284:errorcluster, "Detector de presencia"=w278:bool, "RuedaDetectada1?"=→"RuedaDetectada1?":bool, "RuedaDetectada2?"=→"RuedaDetectada2?":bool)
              n98 = Get Date/Time In Seconds() -> (seconds since 1Jan1904=w280:timestamp)
              n99 = Format Date/Time String(seconds (now)=w280, UTC format=TRUE) -> (date/time string=→"date/time string":string)  [unwired: 1 in]
              n100 = Compound Arithmetic op=OR(w291, w259, w287) -> (w288:bool)
              n101 = case shown="\"Adquirir\"" "Developer commad" {
                tunnel: [w305 w306 FALSE ("Adquirir") FALSE ("Adquirir")] -> w264
                tunnel: [FALSE ("Adquirir") w306 w307 w309] -> w263
                frame "Adquirir" {
                  w305 = TRUE ("Adquirir")
                  "Adquirir" <- w305
                }
                frame Default {
                  w306 = FALSE ("Adquirir")
                }
                frame "STOP_WHD" {
                  w307 = TRUE ("Adquirir")
                  "Parar la aplicación" <- w307
                }
                frame "Reset_Controlador" {
                  w309 = TRUE ("Adquirir")
                  "Reset del controlador" <- w309
                }
              }
              "Boton Adquirir?" <- w264
              n102 = xnode "Read/Write Control"("FPGA VI Reference In"=w285, "error in"=w284, "Fotocélula"=w264) -> ("FPGA VI Reference Out"=w275:refnum<k20>, "error out"=w274:errorcluster)
              n103 = Select(t="TEST", s=w288, f="Adquisición") -> (s? t:f=w300:string)
              n104 = Select(t="Configuración", s=w263, f=w300) -> (s? t:f=w268:string)
              n105 = Compound Arithmetic op=OR(w264, w288, w263, w278, "Calibration", "Diagnosis") -> (w265:bool)
              n106 = Select(t="Calibracion", s="Calibration", f=w268) -> (s? t:f=w254:string)
              n107 = Select(t="Diagnosis", s="Diagnosis", f=w254) -> (s? t:f=w252:string)
              n108 = Select(t="UPS", s=w259, f=w252) -> (s? t:f=w260:string)
              n109 = Equal?(x="Developer password", y="cafdsadmin") -> (x = y?=w256:bool)
              n110 = property on="Value to compare" class="Arr (strict)"("Visible"=w256) -> ()  [unwired: 2 in, 2 out]
              n111 = property on="mean" class="Arr (strict)"("Visible"=w256) -> ()  [unwired: 2 in, 2 out]
              n112 = property on="median" class="Arr (strict)"("Visible"=w256) -> ()  [unwired: 2 in, 2 out]
              n113 = property on="max" class="Arr (strict)"("Visible"=w256) -> ()  [unwired: 2 in, 2 out]
              n114 = property on="min" class="Arr (strict)"("Visible"=w256) -> ()  [unwired: 2 in, 2 out]
              n115 = property on="Waveform Graph" class="WFGraph (strict)"("Visible"=w256) -> ()  [unwired: 2 in, 2 out]
            }
            n116 = call <vilib>:"Watchdog Clear.vi"("error in (no error)"=w227, "watchdogID in"=w228) -> ("error out"=w226:errorcluster)  [unwired: 5 in]
            n117 = xnode "Read/Write Control"("FPGA VI Reference In"=w222, "error in"=w215) -> ("FPGA VI Reference Out"=w221:refnum<k20>, "error out"=w220:errorcluster, "Direccion 0?"=→"Direccion 0?":bool)
            n118 = Unbundle By Name(w220) -> ("status"=w237:bool)
            n119 = Select(t="TEST", s=w237, f=w238) -> (s? t:f=w233:string)
            n120 = flat-sequence {
              tunnel: [w249] -> w232
              tunnel: w233 -> [w249]
              frame #0 {
                n121 = Get Date/Time In Seconds() -> (seconds since 1Jan1904=w250:timestamp)
                n122 = To Double Precision Float(number=w250) -> (double precision float=→"Tiempo":dbl)
                n123 = local write "Developer commad"("" ("Developer commad")) -> ()
                n124 = local write "Adquirir"(FALSE ("Adquirir")) -> ()
              }
            }
          }
          frame "Adquisición" {
            n125 = local read "Watchdog config"() -> (w327:T2)
            n126 = flat-sequence {
              tunnel: w316 -> [w356]
              tunnel: w315 -> [w355]
              tunnel: [w356] -> w314
              tunnel: [w355] -> w313
              frame #0 {
                n127 = local read "Report"() -> (w352:string)
                n128 = call "Reporting_datetime.vi"() -> ("String"=w351:string)  [unwired: 11 in]
                n129 = Concatenate Strings(w351, "\nSTATUS: ACQUISITION\nTrain is passing\n\n", w352) -> (w354:string)
                n130 = local write "Report"(w354) -> ()
              }
            }
            n131 = call <vilib>:"Watchdog Configure.vi"("error in (no error)"=w326, "expiration actions"=w327, "timeout (1 sec)"=200.0) -> ("error out"=w324:errorcluster, "watchdogID"=w325:u64)  [unwired: 1 in, 2 out]
            n132 = flat-sequence {
              tunnel: w313 -> [w390]
              tunnel: w314 -> [w391]
              tunnel: [w389] -> w341
              tunnel: [w388] -> w340
              tunnel: [w387] -> w339
              tunnel: [w386] -> w338
              tunnel: [w385] -> w337
              tunnel: [w384] -> w336
              tunnel: [w374] -> w329
              tunnel: w325 -> [w373]
              tunnel: w324 -> [w372]
              tunnel: [w373] -> w323
              tunnel: [w372] -> w322
              tunnel: [w406] -> w350
              tunnel: [w423] -> w349
              tunnel: [w422] -> w348
              tunnel: [w421] -> w347
              tunnel: [w414] -> w346
              tunnel: w341 -> [w420]
              tunnel: w340 -> [w419]
              tunnel: w339 -> [w418]
              tunnel: w338 -> [w417]
              tunnel: w337 -> [w416]
              tunnel: w336 -> [w415]
              tunnel: w329 -> [w412]
              tunnel: [w411] -> w328
              tunnel: w323 -> [w410]
              tunnel: w322 -> [w409]
              tunnel: [w407] -> w321
              tunnel: w350 -> [w586]
              tunnel: w349 -> [w583]
              tunnel: w348 -> [w582]
              tunnel: w347 -> [w599]
              tunnel: [w621] -> w333
              tunnel: w346 -> [w623]
              tunnel: [w614] -> w343
              tunnel: [w615] -> w345
              tunnel: [w616] -> w344
              tunnel: w328 -> [w595]
              tunnel: w321 -> [w587]
              tunnel: [w587] -> w319
              tunnel: [w586] -> w318
              frame #0 {
                n133 = local read "Offset_rueda WS 1"() -> (w367:fxp<+/-,24,-4>)
                n134 = local read "Offset_rueda WS 2"() -> (w368:fxp<+/-,24,-4>)
                n135 = local read "Frecuencia de muestreo (Hz)"() -> (w382:dbl)
                n136 = local read "Escaneos de la FIFO por canal"() -> (w371:u32)
                n137 = local read "Canal cero WS1?"() -> (w376:bool)
                n138 = local read "Count(mSec)"() -> (w375:u32)
                n139 = local read "Frecuencia de muestreo y módulo CRIO"() -> (w378:T3)
                n140 = local read "Canal cero WS2"() -> (w366:bool)
                n141 = local read "Digital?"() -> (w377:bool)
                n142 = Get Date/Time In Seconds() -> (seconds since 1Jan1904=→"Inicio pasada":timestamp)
                n143 = local read "Nº de acelerómetros"() -> (w364:i32)
                n144 = local read "Nº inductivos"() -> (w365:i32)
                n145 = xnode "Read/Write Control"("FPGA VI Reference In"=w391, "error in"=w390, "Data Rate"=w378, "Digital?"=w377, "Canal cero WS1?"=w376, "Count(mSec)"=w375, "Offset_WS1"=w367, "Offset_WS2"=w368, "Canal cero WS2?"=w366) -> ("FPGA VI Reference Out"=w381:refnum<k20>, "error out"=w380:errorcluster)
                n146 = local read "RFID LR6 on?"() -> (w369:bool)
                n147 = Add(x=w365, y=w364) -> (x+y=w370:i32)
                n148 = case shown="True" w369 {
                  tunnel: [errorcluster {"status"=FALSE, "code"=0, "source"=""} ("error out") w396] -> w374
                  frame False {
                  }
                  frame True {
                    n149 = local read "RFID_LR6_Error"() -> (w397:errorcluster)
                    n150 = call "LH6HD.vi"("error in (no error)"=w397, "Action"=enum16{"Init", "Start", "Read", "Stop", "Exit"}."Start") -> ("error out"=w396:errorcluster)  [unwired: 8 in, 1 out]
                  }
                }
                n151 = call "DMACalc.vi"("Number of Channels"=w370, "Number of Samples"=w371, "Rate (Hz)"=w382) -> ("Block Size"=w386:u32, "Time to Acquire Block (ms)"=w387:i32, "Host Buffer Size"=w392:u32)  [unwired: 6 in]
                n152 = call "Pathhorafech(SubVI)_varios.vi"("Folder path"=path "c:/Trenes", "Nº de acelerómetros"=w364, "Nº inductivos"=w365) -> ("Acel_Paths"=w360:path[])  [unwired: 1 in, 1 out]
                "Nombre de archivo" <- w360
                n153 = Index Array(array=w360) -> (element=w359:path)  [unwired: 1 in]
                n154 = for {
                  tunnel: w360 -> [w401] mode=indexing
                  tunnel: [w400] -> w385 mode=indexing
                  tunnel: [w399] -> w384
                  n155 = Open/Create/Replace File(file path (use dialog)=w401, operation (0:open)=T5."replace or create", access (0:read/write)=enum16{"read/write", "read-only", "write-only"}."read/write", disable buffering (F)=TRUE) -> (refnum out=w400:refnum<file>, error out=w399:errorcluster)  [unwired: 1 in, 2 out]
                }
                n156 = xnode "Invoke Method"("FPGA VI Reference In"=w381, "error in"=w380, "Requested Depth"=w392) -> ("FPGA VI Reference Out"=w394:refnum<k20>, "error out"=w393:errorcluster)  [unwired: 1 out]
                n157 = local read "Report"() -> (w363:string)
                n158 = Path To String(path=w359) -> (string=w357:string)
                n159 = Concatenate Strings("\nFile created: ", w357, "\n", w363) -> (w362:string)
                n160 = xnode "Invoke Method"("FPGA VI Reference In"=w394, "error in"=w393) -> ("FPGA VI Reference Out"=w389:refnum<k20>, "error out"=w388:errorcluster)
                n161 = local write "Report"(w362) -> ()
              }
              frame #1 {
                n162 = while "Data Acquisition" {
                  tunnel: w420 -> [w474]
                  shift-right: [w498] -> _
                  shift-left: u32 0 ("t") -> [w494]
                  tunnel: w418 -> [w499]
                  tunnel: w417 -> [w497]
                  shift-right: [w500] -> w422
                  shift-left: w419 -> [w491]
                  tunnel: [w495] -> w423
                  tunnel: w416 -> [w478]
                  tunnel: [w479] -> w421
                  shift-right: [w477] -> w414
                  shift-left: w415 -> [w487]
                  stop <- w496 stop-if-true
                  # "Detector de presencia"
                  # "Mide el tiempo de paso del tren y con ello se puede calcular\nla velocidad la unidad"
                  n163 = xnode "Invoke Method"("FPGA VI Reference In"=w474, "error in"=w491, "Number of Elements"=w494, "Timeout (ms)"=0) -> ("FPGA VI Reference Out"=w471:refnum<k20>, "error out"=w476:errorcluster, "Data"=w490:fxp<+/-,24,4>[], "Elements Remaining"=w492:u32)
                  n164 = case "Data Ready" shown="Default" w494 {
                    tunnel: w499 -> [w522 _]
                    tunnel: [w521 u32 0 ("t")] -> w498
                    tunnel: w497 -> [w523 _]
                    tunnel: w492 -> [w520 _]
                    tunnel: w490 -> [_ w545]
                    tunnel: w487 -> [w519 w544]
                    tunnel: [w519 w546] -> w477
                    tunnel: w478 -> [w518 w543]
                    tunnel: [w518 w542] -> w479
                    frame 0 {
                      # "En este caso se compara los elementos que quedan\nen la FIFO del controlador con el tamaño dell bloque\nque aparece en el panel frontal. Si el número de \nelementos en la FIFO es mayor o igual que el tamaño\n del bloque se pasa al siguiente caso y se guardan \nlos datos en un archivo. El reloj que aparece es una\nespera para no consumir recursos."
                      n165 = Greater Or Equal?(x=w520, y=w523) -> (x >= y?=w524:bool)
                      n166 = case shown="False" w524 {
                        tunnel: [u32 0 ("Block Size") w528] -> w521
                        tunnel: [w527 0 ("t")] -> w525
                        tunnel: w522 -> [w527 _]
                        tunnel: w523 -> [_ w528]
                        frame False {
                        }
                        frame True {
                        }
                      }
                      n167 = call "WaitMinTimeBetweenCall.vi"("Minimum ms between calls"=w525) -> ()  [unwired: 2 in]
                    }
                    frame Default {
                      n168 = To Single Precision Float(number=w545) -> (single precision float=w532:sgl[])
                      n169 = Decimate 1D Array(w532) -> (w538:sgl[], w541:sgl[], w540:sgl[], w539:sgl[], w537:sgl[], w536:sgl[], w535:sgl[], w534:sgl[], w533:sgl[], w530:sgl[])
                      n170 = Build Array(w538, w541, w540, w539, w537, w536, w535, w534, w533, w530) -> (w531:sgl[][])
                      n171 = for {
                        tunnel: T6."little-endian" ("byte order (0:big-endian, network order)") -> [w555]
                        shift-right: [w549] -> w546
                        shift-left: w544 -> [w550]
                        tunnel: w531 -> [w553] mode=indexing
                        tunnel: w543 -> [w552] mode=indexing
                        tunnel: [w551] -> w542 mode=indexing
                        n172 = Write to Binary File(file (use dialog)=w552, data=w553, error in=w550, 5:FALSE ("prepend array or string size? (T)"), 9:w555) -> (refnum out=w551:refnum<file>, error out=w549:errorcluster)  [unwired: 2 out]
                      }
                    }
                  }
                  n173 = xnode "Read/Write Control"("FPGA VI Reference In"=w471, "error in"=w476) -> ("FPGA VI Reference Out"=w489:refnum<k20>, "error out"=w488:errorcluster, "Parar"=w467:bool, "Nº Ruedas 1"=→"Nº Ruedas 1":i32, "NºRuedas 2"=→"NºRuedas 2":i32)
                  "Parar" <- w467
                  n174 = case shown="False" w467 {
                    tunnel: [w505 w513] -> w468
                    tunnel: [w506 0.0] -> w482
                    frame False {
                      n175 = local read "Inicio pasada"() -> (w509:timestamp)
                      n176 = Get Date/Time In Seconds() -> (seconds since 1Jan1904=w508:timestamp)
                      n177 = local read "Tiempo de adquisicion"() -> (w501:dbl)
                      n178 = To Double Precision Float(number=w508) -> (double precision float=w507:dbl)
                      n179 = To Double Precision Float(number=w509) -> (double precision float=w510:dbl)
                      n180 = Subtract(x=w507, y=w510) -> (x-y=w506:dbl)
                      "Tiempo de paso (s)" <- w506
                      n181 = local write "Tiempo"(w507) -> ()
                      n182 = local read "Boton Adquirir?"() -> (w502:bool)
                      n183 = Greater?(x=w506, y=w501) -> (0:w504:bool)
                      n184 = Select(t=w504, s=w502, f=FALSE) -> (s? t:f=w505:bool)
                    }
                    frame True {
                      n185 = local read "Tiempo"() -> (w517:dbl)
                      n186 = local read "Tiempo extra al detector de paso (s)"() -> (w512:dbl)
                      n187 = Get Date/Time In Seconds() -> (seconds since 1Jan1904=w514:timestamp)
                      n188 = To Double Precision Float(number=w514) -> (double precision float=w515:dbl)
                      n189 = Subtract(x=w515, y=w517) -> (x-y=w516:dbl)
                      n190 = Greater?(x=w516, y=w512) -> (0:w513:bool)
                    }
                  }
                  "Fin" <- w468
                  n191 = local read "Timeout ruedas"() -> (w466:dbl)
                  n192 = xnode ("CheckLate")("FPGA VI Reference In"=w489, "error in"=w488) -> ("FPGA VI Reference Out"=w473:refnum<k20>, "error out"=w484:errorcluster, "Buffer Underflow"=→"Buffer Underflow":bool, "Buffer Overflow"=w475:bool)
                  "Buffer Overflow" <- w475
                  n193 = Greater?(x=w482, y=w466) -> (0:w480:bool)
                  "Timeout ruedas" <- w480
                  n194 = call "ErrorOverFlow.vi"("Buffer Overflow"=w475) -> ("error out"=w483:errorcluster)
                  n195 = Merge Errors(w484, w483) -> (w472:errorcluster)
                  n196 = Unbundle By Name(w477) -> ("status"=w481:bool)
                  n197 = Unbundle By Name(w472) -> ("status"=w486:bool)
                  n198 = Compound Arithmetic op=OR(w486, w468, w480, w481) -> (w496:bool)
                  "result" <- w496
                  n199 = case "Flush" shown="True" w496 {
                    tunnel: [w556 w561] -> w500
                    tunnel: [w557 w560] -> w495
                    tunnel: w473 -> [w557 w559]
                    tunnel: w472 -> [w556 w558]
                    frame False {
                    }
                    frame True {
                      n200 = xnode "Invoke Method"("FPGA VI Reference In"=w559, "error in"=w558) -> ("FPGA VI Reference Out"=w560:refnum<k20>, "error out"=w561:errorcluster)
                    }
                  }
                  "Block Size" <- w497
                  "Time to Acquire Block (ms)" <- w499
                }
                n201 = call <vilib>:"Watchdog Whack.vi"("error in (no error)"=w409, "reset watchdog after expire? (F)"=TRUE, "watchdogID in"=w410) -> ("error out"=w406:errorcluster, "watchdogID out"=w407:u64)  [unwired: 2 in, 1 out]
                n202 = local read "RFID LR6 on?"() -> (w405:bool)
                n203 = case shown="True" w405 {
                  tunnel: w412 -> [w424 w430]
                  tunnel: [w424 w429] -> w411
                  frame False {
                  }
                  frame True {
                    n204 = while {
                      shift-right: [w437] -> w429
                      shift-left: w430 -> [w438]
                      shift-right: [w436] -> w427
                      shift-left: string[] [] -> [w435]
                      shift-right: [w431] -> w425
                      shift-left: i32[] [] -> [w432]
                      i -> [w433]
                      stop <- w434 stop-if-true
                      n205 = case shown="No Error" w438 {
                        selector: w438 -> [w449 _]
                        tunnel: [w448 w464] -> w437
                        tunnel: [w444 string[] []] -> w436
                        tunnel: w435 -> [w443 _]
                        tunnel: w433 -> [w442 _]
                        tunnel: w432 -> [w441 _]
                        tunnel: [w440 i32[] []] -> w431
                        frame No Error {
                          n206 = call "LH6HD.vi"("error in (no error)"=w449, "Action"=enum16{"Init", "Start", "Read", "Stop", "Exit"}."Read") -> ("error out"=w448:errorcluster, "Tag"=w445:string)  [unwired: 8 in]
                          n207 = Not Equal?(x="", y=w445) -> (x != y?=w446:bool)
                          n208 = case shown="False" w446 {
                            tunnel: w445 -> [_ w458]
                            tunnel: [w452 w457] -> w444
                            tunnel: w443 -> [w452 w456]
                            tunnel: w442 -> [_ w453]
                            tunnel: w441 -> [w451 w455]
                            tunnel: [w451 w454] -> w440
                            frame False {
                            }
                            frame True {
                              n209 = Build Array (concatenate)(w456, w458) -> (w457:string[])
                              n210 = Build Array (concatenate)(w455, w453) -> (w454:i32[])
                            }
                          }
                        }
                        frame Error {
                          n211 = local read "LR6 IP address"() -> (w461:string)
                          n212 = local read "DeviceAddress"() -> (w459:u8)
                          n213 = local read "Port LR6"() -> (w462:u16)
                          n214 = call "LH6HD.vi"("DeviceAddress"=w459, "Reader Port"=w462, "IP Address"=w461, "Action"=enum16{"Init", "Start", "Read", "Stop", "Exit"}."Init") -> ("error out"=w464:errorcluster)  [unwired: 6 in, 1 out]
                        }
                      }
                      n215 = Wait Until Next ms Multiple(millisecond multiple=u32 500) -> ()  [unwired: 1 out]
                      n216 = local read "result"() -> (w434:bool)
                      "it-LR6" <- w433
                    }
                    "TAGs LR6" <- w427
                    "it-read-LR6" <- w425
                  }
                }
              }
              frame #2 {
                # "ORGANIZAR\nTAGS AQUÍ"
                n217 = local read "RFID LR6 on?"() -> (w584:bool)
                n218 = local read "RFID NEM on?"() -> (w585:bool)
                n219 = Array Size(array=w599) -> (size(s)=w597:i32)
                n220 = local read "AURA wheel test"() -> (w565:bool)
                n221 = Decrement(x=w597) -> (x-1=w598:i32)
                n222 = case shown="True" w584 {
                  tunnel: w595 -> [w629 w635]
                  tunnel: [w629 w630] -> w594
                  frame False {
                  }
                  frame True {
                    n223 = call "LH6HD.vi"("error in (no error)"=w635, "Action"=enum16{"Init", "Start", "Read", "Stop", "Exit"}."Stop") -> ("error out"=w630:errorcluster)  [unwired: 8 in, 1 out]
                    n224 = call "Reporting_error.vi"("error out 2"=w630, "Concept"="Active RFID") -> ("Reporting"=w632:string)  [unwired: 1 in]
                    n225 = local read "Report"() -> (w633:string)
                    n226 = Concatenate Strings(w632, w633) -> (w631:string)
                    n227 = local write "Report"(w631) -> ()
                  }
                }
                n228 = case shown="True" w585 {
                  tunnel: [string[] [] ("TagArray") w642] -> w563
                  tunnel: [cluster{"TagCode":string, "FirstSeemUs":u64}[] [] ("TagData out") w641] -> w562
                  frame False {
                  }
                  frame True {
                    n229 = call "IF2_TagBuffer.vi"("Action"=enum16{"Init", "WriteTagData", "ReadTagData"}."ReadTagData") -> ("error out"=w640:errorcluster, "TagData out"=w641:cluster{"TagCode":string, "FirstSeemUs":u64}[])  [unwired: 9 in]
                    n230 = local read "connection ID"() -> (w639:refnum<k5>)
                    n231 = call "RFID_TAGS_Sort.vi"("TagData in"=w641) -> ("TagString"=w643:string, "TagArray"=w642:string[])  [unwired: 9 in]
                    n232 = call "IF2_Clear_buffer.vi"("error in (no error)"=w640, "TCP Network Connection in"=w639) -> ()  [unwired: 8 in, 2 out]
                    n233 = call "Reporting_error.vi"("error out 2"=w640, "Concept explanation"=w643, "Concept"="Passive RFID") -> ("Reporting"=w646:string)
                    n234 = local read "Report"() -> (w647:string)
                    n235 = Concatenate Strings(w646, w647) -> (w645:string)
                    n236 = local write "Report"(w645) -> ()
                  }
                }
                "TAGs HEX" <- w563
                n237 = Index Array(array=w599, index=w598) -> (element=w607:refnum<file>)
                n238 = local write "result"(FALSE ("result")) -> ()
                n239 = xnode "Read/Write Control"("FPGA VI Reference In"=w583, "error in"=w582) -> ("FPGA VI Reference Out"=w620:refnum<k20>, "error out"=w580:errorcluster, "Chassis Temperature"=w628:i16)
                n240 = local read "TAGs LR6"() -> (w567:string[])
                n241 = Select(t=string[] ["A0000000000000000TESTNEM7", "A0000000000000000TESTNEM8"], s=w565, f=w567) -> (s? t:f=w564:string[])
                n242 = Divide(x=w628, y=4.0) -> (x/y=w576:dbl)
                "Temperatura (ºC)" <- w576
                n243 = local read "Tiempo de paso (s)"() -> (w618:dbl)
                n244 = for {
                  tunnel: w564 -> [w651] mode=indexing
                  tunnel: [w649] -> w588 mode=indexing
                  n245 = Search and Replace String(input string=w651, search string="00") -> (result string=w649:string)  [unwired: 6 in, 3 out]
                }
                n246 = local write "RFID_LR6_Error"(w594) -> ()
                n247 = Index Array(array=w563) -> (element=w593:string)  [unwired: 1 in]
                n248 = local read "Nº Ruedas 1"() -> (w574:i32)
                n249 = local read "NºRuedas 2"() -> (w578:i32)
                n250 = Not Equal?(x=w593, y="" ("delimiter (\\t)")) -> (x != y?=w591:bool)
                "Plataformas?" <- w591
                n251 = Multiply(x=w618, y=1000.0) -> (x*y=w575:dbl)
                n252 = case shown="True" w591 {
                  tunnel: w588 -> [w652 w659]
                  tunnel: [w652 w658] -> w577
                  tunnel: w563 -> [_ _]
                  tunnel: w562 -> [_ w654]
                  frame False {
                  }
                  frame True {
                    n253 = local read "Tiempo de paso (s)"() -> (w657:dbl)
                    n254 = local read "Tabla_flota"() -> (w655:string[][])
                    n255 = local read "Inicio pasada"() -> (w656:timestamp)
                    n256 = local read "RFID_status"() -> (w653:path)
                    n257 = call "Union_TAGs_RFIDs.vi"("TAGs LR6"=w659) -> ()  [unwired: 1 in, 1 out]
                    n258 = call "write_tag_status.vi"("Inicio pasada"=w656, "Tabla_flota"=w655, "TagData in"=w654, "file path (use dialog)"=w653) -> ()  [unwired: 7 in]
                    n259 = call "TagNormalizaction.vi"("Inicio pasada"=w656, "Tiempo de paso (s)"=w657, "TagData in"=w654, "Tabla_flota"=w655) -> ("Normalized Tags"=w658:string[])  [unwired: 7 in]
                  }
                }
                "TAGs" <- w577
                n260 = Build Array(w576, w575, w574, w578) -> (w579:dbl[])
                n261 = Build Array(w576, w575, w574) -> (w573:dbl[])
                n262 = local read "Direccion 0?"() -> (w572:bool)
                n263 = local read "Nombre de archivo"() -> (w606:path[])
                n264 = Bundle("error out"=w580, w579, "Normalized Tags"=w577, "Direccion 0?"=w572) -> (w571:T11)  [unwired: 1 in]
                n265 = for {
                  shift-right: [w665] -> w612
                  shift-left: string[] [] -> [w664]
                  tunnel: w577 -> [w663] mode=indexing
                  n266 = Insert Into Array(array=w664, new element=w663) -> (w665:string[])  [unwired: 1 in]
                }
                n267 = xnode "Read/Write Control"("FPGA VI Reference In"=w620, "error in"=w580, "Stop"=TRUE ("stop")) -> ("FPGA VI Reference Out"=w609:refnum<k20>, "error out"=w608:errorcluster)
                n268 = call "Reporting_acqu.vi"("output cluster"=w571, "address repoting"=path "C:/Reporting/Reporting_adqu.txt" ("file (use dialog)")) -> ("Reporting"=w568:string)  [unwired: 1 in]
                n269 = Delete From Array(array=w606) -> (deleted portion=w605:path)  [unwired: 2 in, 1 out]
                n270 = local read "Report"() -> (w569:string)
                n271 = To Single Precision Float(number=w573) -> (single precision float=w626:sgl[])
                n272 = Path To String(path=w605) -> (string=w611:string)
                n273 = Concatenate Strings(w568, w569) -> (w570:string)
                n274 = Write to Binary File(file (use dialog)=w607, data=w626, error in=w623, 5:FALSE ("prepend array or string size? (T)"), 9:T6."little-endian" ("byte order (0:big-endian, network order)")) -> (error out=w604:errorcluster)  [unwired: 3 out]
                n275 = xnode "Invoke Method"("FPGA VI Reference In"=w609, "error in"=w608) -> ("FPGA VI Reference Out"=w616:refnum<k20>, "error out"=w615:errorcluster)
                n276 = local read "Timeout ruedas"() -> (w619:bool)
                n277 = local write "Report"(w570) -> ()
                n278 = Build Array (concatenate)(w611, w612) -> (w589:string[])
                n279 = local read "TAGS leidos"() -> (w600:path)
                n280 = for {
                  shift-right: [w662] -> w614
                  shift-left: w604 -> [w661]
                  tunnel: w599 -> [w660] mode=indexing
                  n281 = Close File(refnum=w660, error in=w661) -> (error out=w662:errorcluster)  [unwired: 1 out]
                }
                n282 = call-poly <vilib>:"Write Delimited Spreadsheet.vi"("file path (dialog if empty)"=w600, "1D data"=w589, "append to file? (F)"=TRUE ("transpose? (no:F)"), "transpose? (F)"=TRUE ("append to file? (new file:F)"), "delimiter (\\t)"=";" ("delimiter (\\t)")) -> ()  [unwired: 9 in, 2 out]
                n283 = Select(t="TEST", s=w619, f="Procesado") -> (s? t:f=w621:string)
              }
            }
            n284 = call <vilib>:"Watchdog Clear.vi"("error in (no error)"=w318, "watchdogID in"=w319) -> ("error out"=w320:errorcluster)  [unwired: 5 in]
            n285 = Unbundle By Name(w345) -> ("status"=w334:bool)
            n286 = Unbundle By Name(w343) -> ("status"=w335:bool)
            n287 = Merge Errors(w343, w320) -> (w342:errorcluster)
            n288 = Compound Arithmetic op=OR(w334, w335) -> (w332:bool)
            n289 = Select(t="TEST", s=w332, f=w333) -> (s? t:f=w330:string)
          }
          frame "Procesado" {
            n290 = local read "Watchdog config"() -> (w677:T2)
            n291 = flat-sequence {
              tunnel: w671 -> [w690]
              tunnel: [w690] -> w670
              tunnel: w669 -> [w686]
              tunnel: [w686] -> w668
              frame #0 {
                n292 = local read "Report"() -> (w687:string)
                n293 = call "Reporting_datetime.vi"() -> ("String"=w685:string)  [unwired: 11 in]
                n294 = Concatenate Strings(w685, "\nSTATUS: PROCESSING\nProcessing the measurement\n\n", w687) -> (w689:string)
                n295 = local write "Report"(w689) -> ()
              }
            }
            n296 = call <vilib>:"Watchdog Configure.vi"("error in (no error)"=w680, "expiration actions"=w677, "timeout (1 sec)"=300.0) -> ("error out"=w679:errorcluster, "watchdogID"=w676:u64)  [unwired: 1 in, 2 out]
            n297 = flat-sequence {
              tunnel: w679 -> [w697]
              tunnel: w676 -> [w693]
              tunnel: [w692] -> w675
              tunnel: [w691] -> w674
              tunnel: [w908] -> w673
              tunnel: w675 -> [w908]
              tunnel: [w907] -> w672
              tunnel: w674 -> [w907]
              frame #0 {
                n298 = flat-sequence {
                  tunnel: [w769] -> w699
                  tunnel: [w755] -> w698
                  tunnel: w697 -> [w736]
                  tunnel: [w718] -> w694
                  tunnel: [w757] -> w696
                  tunnel: [w709] -> w695
                  tunnel: w693 -> [w737]
                  tunnel: [w734] -> w692
                  tunnel: [w733] -> w691
                  frame #0 {
                    n299 = local read "AURA wheel test"() -> (w707:bool)
                    n300 = case shown="False" w707 {
                      tunnel: [w772 w773] -> w706
                      tunnel: [w771 path[] [path "c:/Trenes_prueba/A_0_TEST.bin", path "c:/Trenes_prueba/A_1_TEST.bin", path "c:/Trenes_prueba/A_2_TEST.bin", path "c:/Trenes_prueba/A_3_TEST.bin", path "c:/Trenes_prueba/A_4_TEST.bin", path "c:/Trenes_prueba/A_5_TEST.bin", path "c:/Trenes_prueba/A_6_TEST.bin", path "c:/Trenes_prueba/A_7_TEST.bin", path "c:/Trenes_prueba/I_0_TEST.bin", path "c:/Trenes_prueba/I_1_TEST.bin"]] -> w705
                      frame False {
                        n301 = local read "Nombre de archivo"() -> (w771:path[])
                        n302 = local read "TAGs"() -> (w772:string[])
                      }
                      frame True {
                        w773 = string[] ["A0000000000000000TESTNEM7", "A0000000000000000TESTNEM8"]
                        n303 = local write "TAGs LR6"(w773) -> ()
                      }
                    }
                    n304 = local read "Tabla_flota"() -> (w754:string[][])
                    n305 = call <vilib>:"Watchdog Whack.vi"("error in (no error)"=w736, "reset watchdog after expire? (F)"=TRUE, "watchdogID in"=w737) -> ("error out"=w733:errorcluster, "watchdogID out"=w734:u64)  [unwired: 2 in, 1 out]
                    n306 = local read "Puntos medios de las ventanas"() -> (w756:dbl[][])
                    n307 = call "Series_ejes_flota.vi"("Tabla_flota"=w754, "Tags"=w706) -> ("Nº Ejes"=w731:i32[], "Series del convoy"=w748:string[])  [unwired: 2 in, 1 out]
                    "Nº Ejes" <- w731
                    n308 = Array Size(array=w705) -> (size(s)=w763:i32)
                    n309 = Add Array Elements(numeric array=w731) -> (sum=w717:i32)
                    "Ejes_convoy" <- w717
                    n310 = Subtract(x=w763, y=2 ("length")) -> (x-y=w765:i32)
                    n311 = Array Size(array=w748) -> (size(s)=→"Nº UTs":i32)
                    n312 = local read "Series_flota"() -> (w753:string[])
                    n313 = Delete From Array(array=w705, length=2, index=w765) -> (deleted portion=w738:path[], array with subset deleted=w757:path[])
                    n314 = Index Array(array=w738) -> (element #2=w732:path)  [unwired: 2 in, 1 out]
                    n315 = call "Distancias_ejes_convoy.vi"("Series_flota1"=w748, "Ejes_UT"=w731, "Puntos medios de las ventanas"=w756, "Series_flota"=w753) -> ("Distancias_entre_ejes_convoy"=w755:dbl[])  [unwired: 1 in]
                    n316 = Read from Binary File(5:sgl 0.0, 9:T6."little-endian" ("byte order (0:big-endian, network order)"), 10:-1 ("count (1)"), 11:w732) -> (0:w761:errorcluster, 2:w740:sgl[], 3:w762:refnum<file>)  [unwired: 1 in, 2 out]
                    n317 = local read "Frecuencia de muestreo (Hz)"() -> (w722:dbl)
                    n318 = local read "Offset_rueda WS 2"() -> (w723:fxp<+/-,24,-4>)
                    n319 = local read "it-LR6"() -> (w743:i32)
                    n320 = local read "it-read-LR6"() -> (w744:i32[])
                    n321 = local read "Plataformas?"() -> (w742:bool)
                    n322 = local read "TAGs"() -> (w746:string[])
                    n323 = local read "TAGs LR6"() -> (w745:string[])
                    n324 = Close File(refnum=w762, error in=w761) -> (error out=w701:errorcluster)  [unwired: 1 out]
                    n325 = Array Size(array=w740) -> (size(s)=w752:i32)
                    n326 = Subtract(x=w752, y=3 ("length")) -> (x-y=w750:i32)
                    n327 = Delete From Array(array=w740, length=3, index=w750) -> (array with subset deleted=w729:sgl[])  [unwired: 1 out]
                    n328 = call "TAGs_AURAwheel_TAGM_NEM.vi"("Nº Ejes"=w731, "TAGs"=w746, "Ejes_convoy"=w717, "it-LR6"=w743, "TAGs LR6"=w745, "it-read-LR6"=w744, "Plataformas?"=w742) -> ("TAGS_AURA"=→"TAGs_AURAwheel":string[][])  [unwired: 1 in]
                    n329 = call "Analogico_digital.vi"("Array"=w729, "Offset WS"=w723, "Frecuencia muestreo"=w722) -> ("array w/ subset deleted"=w724:sgl[], "Tiempo\npaso"=w721:dbl)  [unwired: 6 in]
                    n330 = call "Puntos medio de pulso.vi"("DI Inductivo"=w724) -> ("Puntos"=w769:sgl[], "Número de ejes"=w711:i32)  [unwired: 1 in]
                    "Número de ejes detectados" <- w711
                    n331 = disable-structure shown="Enabled" {
                      disable-tunnel: w729 -> [w781 w784]
                      disable-tunnel: [FALSE ("element") TRUE ("element")] -> w726
                      disable-tunnel: [w775 w783] -> w725
                      frame Disabled {
                        n332 = Equal?(x=w781, y=0.0) -> (x = y?=w778:bool[])
                        n333 = Equal?(x=w781, y=1.0) -> (x = y?=w779:bool[])
                        n334 = Or(x=w778, y=w779) -> (x .or. y?=w775:bool[])
                      }
                      frame Enabled {
                        n335 = Greater?(x=w784, y=0.1) -> (0:w783:bool[])
                      }
                    }
                    n336 = Decrement(x=w711) -> (x-1=w768:i32)
                    n337 = call "Reporting_error.vi"("error out 2"=w701, "Concept"="Measurement reading") -> ("Reporting"=w703:string)  [unwired: 1 in]
                    n338 = Get Volume Info(11:path "c:/" ("path")) -> (1:w712:i64)  [unwired: 1 in, 5 out]
                    "Disco Duro Disponible (bytes)" <- w712
                    n339 = local read "Report"() -> (w704:string)
                    n340 = call "Calculo_Velocidad.vi"("Tiempo de paso (s)"=w721, "Ejes"=w768, "Puntos iniciales de las ventanas"=w755) -> ("V (m/s)"=→"V (m/s)":dbl, "Longitud de la unidad"=→"Longitud de la unidad":dbl)
                    n341 = Concatenate Strings(w703, w704) -> (w702:string)
                    n342 = Equal?(x=w717, y=w711) -> (x = y?=w709:bool)
                    n343 = Not Equal?(x=w711, y=0) -> (x != y?=w708:bool)
                    n344 = Search 1D Array(1D array=w725, element=w726) -> (index of element=w727:i32)  [unwired: 1 in]
                    n345 = local write "Report"(w702) -> ()
                    n346 = Build Array(w717, w711, w712) -> (w716:i64[])
                    n347 = Equal?(x=w727, y=-1) -> (x = y?=w730:bool)
                    n348 = Compound Arithmetic op=AND(w709, w708, w730) -> (w718:bool)
                    "Archivo\nvalido?" <- w718
                    n349 = Bundle(w716, w718) -> (w714:cluster{i64[], bool})  [unwired: 1 in]
                    n350 = call "Reporting_proc.vi"("output cluster 2"=w714, "address repoting"=path "C:/Reporting/Reporting_proc.txt" ("file (use dialog)")) -> ("Reporting"=w713:string)  [unwired: 1 in]
                    n351 = local read "Report"() -> (w719:string)
                    n352 = Concatenate Strings(w713, w719) -> (w720:string)
                    n353 = local write "Report"(w720) -> ()
                  }
                }
                n354 = case shown="True" w694 {
                  tunnel: w699 -> [_ w819]
                  tunnel: w698 -> [_ w817]
                  tunnel: w696 -> [_ w818]
                  tunnel: w695 -> [w786 _]
                  frame False {
                    n355 = local read "Nombre de archivo"() -> (w787:path[])
                    n356 = for {
                      tunnel: w787 -> [w789] mode=indexing
                      tunnel: w786 -> [w788]
                      n357 = flat-sequence {
                        tunnel: w789 -> [w799]
                        tunnel: [w799] -> w792
                        tunnel: [w798] -> w791
                        tunnel: w788 -> [w797]
                        tunnel: w792 -> [w806]
                        tunnel: [w805] -> w790
                        tunnel: w791 -> [w805]
                        tunnel: w790 -> [w808]
                        frame #0 {
                          w798 = path "c:/Est_Adq.csv" ("file path (use dialog)")
                          n358 = Path To String(path=w799) -> (string=w800:string)
                          n359 = Select(t="Nº Ejes detectados WS diferente a Nº Ejes TAGs" ("delimiter (\\t)"), s=w797, f="La señal del inductivo no es digital" ("delimiter (\\t)")) -> (s? t:f=w794:string)
                          n360 = Build Array(w800, w794) -> (w793:string[])
                          n361 = call-poly <vilib>:"Write Delimited Spreadsheet.vi"("file path (dialog if empty)"=w798, "1D data"=w793, "append to file? (F)"=FALSE ("transpose? (no:F)"), "transpose? (F)"=TRUE ("append to file? (new file:F)"), "delimiter (\\t)"=";" ("delimiter (\\t)")) -> ()  [unwired: 9 in, 2 out]
                        }
                        frame #1 {
                          n362 = local read "Borrar archivos\nadquisicion con error"() -> (w804:bool)
                          n363 = case shown="True" w804 {
                            tunnel: w806 -> [_ w807]
                            frame False {
                            }
                            frame True {
                              n364 = Delete(path (use dialog)=w807) -> ()  [unwired: 1 in, 6 out]
                            }
                          }
                        }
                        frame #2 {
                          n365 = File/Directory Info(path=w808) -> (size=w811:i64)  [unwired: 1 in, 6 out]
                          n366 = Greater?(x=w811, y=i64 1000000) -> (0:w809:bool)
                          n367 = case shown="True" w809 {
                            tunnel: w808 -> [_ w812]
                            frame False {
                            }
                            frame True {
                              n368 = Delete(path (use dialog)=w812) -> ()  [unwired: 4 in, 3 out]
                            }
                          }
                        }
                      }
                    }
                  }
                  frame True {
                    n369 = flat-sequence {
                      tunnel: w819 -> [w896]
                      tunnel: w818 -> [w893]
                      tunnel: w817 -> [w897]
                      tunnel: [w880] -> w816
                      frame #0 {
                        # "SALIDA \n\nMáximos por rueda inductivo"
                        # "8 acelerómetros"
                        # "Velocidad"
                        n370 = local read "Frecuencia de muestreo (Hz)"() -> (w895:dbl)
                        n371 = local read "Distancia de acelerómetros"() -> (w885:dbl[])
                        n372 = local read "Parámetros acelerómetros"() -> (w892:dbl[])
                        n373 = local read "Número de ejes detectados"() -> (w891:i32)
                        n374 = local read "Distancias generales"() -> (w890:dbl[])
                        n375 = local read "dt RMS"() -> (w894:dbl)
                        n376 = local read "Direccion 0?"() -> (w882:bool)
                        n377 = Index Array(array=w890, index=1) -> (element=w888:dbl)
                        n378 = Select(t=0.0, s=w882, f=w888) -> (s? t:f=w886:dbl)
                        n379 = Subtract(x=w886, y=w885) -> (x-y=w884:dbl[])
                        n380 = Absolute Value(x=w884) -> (abs(x)=w883:dbl[])
                        n381 = call "Procesado_aRMS_BIdirecc.vi"("Paths_canales_aRMS"=w893, "Ejes Procesados"=w891, "Distancias\nacelerometros"=w883, "Distancias generales (m)"=w890, "Distancias centrales de las ruedas\n               configuración (m)"=w897, "Frecuencia de muestreo"=w895, "Parámetros acelerómetros"=w892, "dt RMS 2"=w894, "Puntos"=w896) -> ("Max RMS Ruedas"=w881:dbl[][])  [unwired: 2 in]
                        n382 = Transpose 2D Array(2D array=w881) -> (transposed array=w880:dbl[][])
                        "Max RMS Ruedas" <- w880
                        n383 = call "Reporting_proc_RMS.vi"("Max RMS Ruedas"=w880) -> ("String"=w878:string)
                        n384 = local read "Report"() -> (w879:string)
                        n385 = Concatenate Strings(w878, w879) -> (w877:string)
                        n386 = local write "Report"(w877) -> ()
                      }
                    }
                    n387 = local read "Use Aura?"() -> (w815:bool)
                    n388 = local read "TAGs_AURAwheel"() -> (w814:string[][])
                    n389 = local read "Nº Ejes"() -> (w813:i32[])
                    n390 = for {
                      tunnel: w815 -> [w823]
                      tunnel: w814 -> [w822] mode=indexing
                      shift-right: [w821] -> _
                      shift-left: w816 -> [w824]
                      tunnel: w813 -> [w820] mode=indexing
                      # "dev.api.aurawheel.com"
                      n391 = case shown="True" w823 {
                        tunnel: w824 -> [w825 w844]
                        tunnel: w822 -> [_ w845]
                        tunnel: [w825 w843] -> w821
                        tunnel: w820 -> [_ w841]
                        frame False {
                        }
                        frame True {
                          w829 = "\n"
                          w852 = cluster{"status":string} {"status"=""}
                          n392 = local read "Parametros AuraWheel"() -> (w876:string[])
                          n393 = Delete From Array(array=w844, length=w841, index (row)=0) -> (deleted portion=w840:dbl[][], array with subset deleted=w843:dbl[][])  [unwired: 1 in]
                          n394 = Get Date/Time In Seconds() -> (seconds since 1Jan1904=w873:timestamp)
                          n395 = Format Date/Time String(time format string (%c)="%H:%M:%S%3u", seconds (now)=w873) -> (date/time string=w871:string)  [unwired: 1 in]
                          n396 = Get Date/Time In Seconds() -> (seconds since 1Jan1904=w848:timestamp)
                          n397 = Scan From String(format string="%d:%d:%f", input string=w871) -> (output 1=w868:i32, output 2=w867:i32, output 3=w865:dbl)  [unwired: 5 in, 3 out]
                          n398 = local read "V (m/s)"() -> (w836:dbl)
                          n399 = local read "Temperatura (ºC)"() -> (w846:dbl)
                          n400 = Multiply(x=w836, y=3.6) -> (x*y=w834:dbl)
                          n401 = Multiply(x=w865, y=1000.0) -> (x*y=w861:dbl)
                          n402 = call "Time_to_ms.vi"("seconds since 1Jan1904"=w848) -> ("Numeric"=w847:dbl)  [unwired: 1 in]
                          n403 = Multiply(x=w867, y=60000) -> (x*y=w862:i32)
                          n404 = Multiply(x=3600000, y=w868) -> (x*y=w863:i32)
                          n405 = Index Array(array=w876) -> (element #1=w839:string, element #2=w838:string, element #3=w837:string)  [unwired: 3 in]
                          n406 = call "aw_WRDCluster_8acel.vi"("Array TAGs"=w845, "Max RMS Ruedas"=w840, "TimeStamp"=w847, "p_sp"=w834, "p_tp"=w846) -> ("JSON cluster"=w874:T12)  [unwired: 1 in]
                          n407 = Compound Arithmetic op=ADD(w863, w862, w861) -> (w860:dbl)
                          n408 = To Variant(anything=w874) -> (Variant=w857:variant)
                          n409 = To Unsigned Long Integer(number=w860) -> (unsigned 32bit integer=w859:u32)
                          n410 = call "gjson_Create.vi"("JSON Object in"=w857) -> ("error out"=w855:errorcluster, "JSON String Out"=w856:string)  [unwired: 9 in]
                          n411 = Number To Decimal String(number=w859) -> (decimal integer string=w858:string)  [unwired: 1 in]
                          n412 = To Variant(anything=w852) -> (Variant=w851:variant)
                          n413 = call "aw_SendData.vi"("pwd"=w839, "x-nem-datetime"=w858, "User"=w838, "error in"=w855, "JSON Object"=w856, "URL"=w837) -> ("error out"=w853:errorcluster, "Response JSON"=w854:string, "Response headers"=w830:string)  [unwired: 3 in]
                          "Response headers" <- w830
                          n414 = call "gjson_Parse.vi"("error in"=w853, "JSON String In"=w854, "JSON Cluster"=w851) -> ("error out"=w849:errorcluster, "JSON Cluster Out"=w850:variant)  [unwired: 7 in]
                          n415 = Variant To Data(error in=w849, type=w852, Variant=w850) -> (data=→"data":cluster{"status":string}, error out=w831:errorcluster)
                          "error AURA" <- w831
                          n416 = local read "Report"() -> (w827:string)
                          n417 = call "Reporting_error.vi"("error out 2"=w831, "Concept"="A.U.R.A. Wheel Connection") -> ("Reporting"=w832:string)  [unwired: 1 in]
                          n418 = Concatenate Strings(w832, w829, w829, w830, w829) -> (w828:string)
                          "Report_AURA" <- w828
                          n419 = Concatenate Strings(w828, w827) -> (w826:string)
                          n420 = local write "Report"(w826) -> ()
                        }
                      }
                    }
                  }
                }
              }
              frame #1 {
                n421 = local read "Archivo\nvalido?"() -> (w904:bool)
                n422 = local read "Bytes libre despues de borrar"() -> (w905:u32)
                n423 = local read "Report_AURA"() -> (w901:string)
                n424 = local read "Max archivos"() -> (w902:u32)
                n425 = local read "Path LOG"() -> (w903:path)
                n426 = local read "LOG.txt"() -> (w898:path)
                n427 = local read "Report"() -> (w900:string)
                n428 = local read "Bytes min libre"() -> (w906:u32)
                n429 = local read "TAGS leidos"() -> (w909:path)
                n430 = File/Directory Info(path=w909) -> (size=w912:i64)  [unwired: 1 in, 6 out]
                n431 = case shown="True" w904 {
                  frame False {
                  }
                  frame True {
                    n432 = local read "Nombre de archivo"() -> (w914:path[])
                    n433 = call "Comprimir_a_1_archivo.vi"("Acel_paths"=w914) -> ("path_Pasada"=→"created path":path)
                  }
                }
                n434 = Greater?(x=w912, y=i64 1000000) -> (0:w910:bool)
                n435 = case shown="True" w910 {
                  tunnel: w909 -> [_ w915]
                  frame False {
                  }
                  frame True {
                    n436 = Delete(path (use dialog)=w915) -> ()  [unwired: 4 in, 3 out]
                  }
                }
                n437 = call "BORRADO_MEJORADO_Gonzalo.vi"("Bytes LIBRE OK"=w905, "Bytes Minimo de Memoria libre"=w906) -> ()  [unwired: 10 in]
                n438 = call "Saving_LOG.vi"("Path"=w898, "Report"=w900, "Report AURA"=w901, "Path Carpeta"=w903, "Nº Archivos Max"=w902) -> ("Report"=w899:string)  [unwired: 9 in, 1 out]
                n439 = local write "Report"(w899) -> ()
              }
            }
            n440 = call <vilib>:"Watchdog Clear.vi"("error in (no error)"=w672, "watchdogID in"=w673) -> ("error out"=w666:errorcluster)  [unwired: 5 in]
            n441 = Merge Errors(w668, w666) -> (w684:errorcluster)
            n442 = Unbundle By Name(w684) -> ("status"=w682:bool)
            n443 = Select(t="TEST", s=w682, f="Espera") -> (s? t:f=w681:string)
          }
          frame "TEST" {
            n444 = flat-sequence {
              tunnel: [w931] -> w918
              tunnel: w920 -> [w931]
              frame #0 {
                n445 = local read "Report"() -> (w932:string)
                n446 = call "Reporting_datetime.vi"() -> ("String"=w930:string)  [unwired: 11 in]
                n447 = Concatenate Strings(w930, "\nSTATUS: ERROR TEST\n\n", w932) -> (w934:string)
                n448 = local write "Report"(w934) -> ()
              }
            }
            n449 = local read "Watchdog config"() -> (w925:T2)
            n450 = Merge Errors(w918, w916) -> (w917:errorcluster)
            n451 = call <vilib>:"Watchdog Configure.vi"("error in (no error)"=w916, "expiration actions"=w925, "timeout (1 sec)"=200.0) -> ("error out"=w926:errorcluster, "watchdogID"=w923:u64)  [unwired: 1 in, 2 out]
            n452 = flat-sequence {
              tunnel: [w944] -> w929
              tunnel: w926 -> [w939]
              tunnel: w917 -> [w957]
              tunnel: [w940] -> w927
              tunnel: w923 -> [w938]
              tunnel: [w937] -> w922
              tunnel: [w936] -> w921
              frame #0 {
                n453 = Get Date/Time In Seconds() -> (seconds since 1Jan1904=w951:timestamp)
                n454 = local read "Ultimo TEST"() -> (w952:timestamp)
                n455 = To Double Precision Float(number=w951) -> (double precision float=w953:dbl)
                n456 = Subtract(x=w953, y=3600.0) -> (x-y=w955:dbl)
                n457 = To Time Stamp(1:w955) -> (0:w956:timestamp)
                n458 = call <vilib>:"Watchdog Whack.vi"("error in (no error)"=w939, "reset watchdog after expire? (F)"=TRUE, "watchdogID in"=w938) -> ("error out"=w936:errorcluster, "watchdogID out"=w937:u64)  [unwired: 2 in, 1 out]
                n459 = In Range and Coerce(upper limit=w951, x=w952, lower limit=w956) -> (In Range?=w950:bool)  [unwired: 1 out]
                n460 = case shown="False" w950 {
                  tunnel: w957 -> [w967 w991]
                  tunnel: [w967 w991] -> w940
                  frame False {
                    n461 = local read "Timeout ruedas"() -> (w968:bool)
                    n462 = local read "Aviso no detección"() -> (w971:string)
                    n463 = local read "Aviso temperatura"() -> (w970:string)
                    n464 = case shown="True" w968 {
                      selector: w968 -> [_ w988]
                      tunnel: ["\r" w989] -> w966
                      frame False {
                      }
                      frame True {
                        w978 = "\n"
                        n465 = local read "Nº Ruedas 1"() -> (w985:i32)
                        n466 = local read "NºRuedas 2"() -> (w980:i32)
                        n467 = call "ErrorRuedas.vi"("Buffer Overflow"=w988) -> ("error out"=w990:errorcluster)
                        n468 = Number To Decimal String(number=w985) -> (decimal integer string=w983:string)  [unwired: 1 in]
                        n469 = Number To Decimal String(number=w980) -> (decimal integer string=w979:string)  [unwired: 1 in]
                        n470 = Concatenate Strings("Error Wheel sensors", "\n", "WS1 (wheels):", w983, w978, "WS2 (wheels):", w979, w978) -> (w981:string)
                        n471 = call "Error.vi"("Error con..."=w981, "error comunicacion 2"=w990) -> ("String"=w989:string)
                      }
                    }
                    n472 = local read "DC OK"() -> (w969:string)
                    n473 = call "Cabecera.vi"() -> ("String"=w976:string)
                    n474 = call "Adquisicion.vi"("Aviso no detección"=w971) -> ("String"=w975:string)
                    n475 = call "Temperatura.vi"("Aviso temperatura"=w970) -> ("String"=w974:string)
                    n476 = call "Fuente.vi"("DC OK"=w969) -> ("String"=w973:string)
                    n477 = call "FPGA.vi"("error out"=w967) -> ("String"=w972:string)
                    n478 = Get Date/Time In Seconds() -> (seconds since 1Jan1904=→"Ultimo TEST":timestamp)
                    n479 = Concatenate Strings(w976, w975, w974, w973, w972, w966) -> (w960:string)
                    n480 = local read "Report"() -> (w959:string)
                    n481 = Concatenate Strings(w960, w959) -> (w961:string)
                    n482 = local read "Max archivos"() -> (w962:u32)
                    n483 = local read "Path LOG"() -> (w965:path)
                    n484 = local read "LOG.txt"() -> (w963:path)
                    n485 = call "Saving_LOG.vi"("Path"=w963, "Report"=w961, "Report AURA"=w960, "Path Carpeta"=w965, "Nº Archivos Max"=w962) -> ("Report"=w964:string)  [unwired: 9 in, 1 out]
                    n486 = local write "Report"(w964) -> ()
                  }
                  frame True {
                  }
                }
                n487 = local read "Fallo fotocelula"() -> (w943:bool)
                n488 = local read "T fuera rango"() -> (w949:bool)
                n489 = Unbundle By Name(w940) -> ("status"=w941:bool)
                n490 = Compound Arithmetic op=OR(w941, w943) -> (w942:bool)
                n491 = local write "Reset del controlador"(w942) -> ()
                n492 = Select(t="UPS", s=w949, f="Espera") -> (s? t:f=w946:string)
                n493 = Select(t="Configuracion", s=w942, f=w946) -> (s? t:f=w944:string)
              }
            }
            n494 = call <vilib>:"Watchdog Clear.vi"("error in (no error)"=w921, "watchdogID in"=w922) -> ("error out"=w919:errorcluster)  [unwired: 5 in]
          }
          frame "Calibracion" {
            n495 = flat-sequence {
              tunnel: w1007 -> [w1792]
              tunnel: w1006 -> [w1791]
              tunnel: [w1792] -> w1005
              tunnel: [w1791] -> w1004
              frame #0 {
                n496 = local read "Report"() -> (w1788:string)
                n497 = call "Reporting_datetime.vi"() -> ("String"=w1787:string)  [unwired: 11 in]
                n498 = Concatenate Strings(w1787, "\nSTATUS: CALIBRATION\n\n\n", w1788) -> (w1790:string)
                n499 = local write "Report"(w1790) -> ()
              }
            }
            n500 = for {
              N: 5 -> [_]
              shift-right: [w1046] -> w998
              shift-left: w1005 -> [w1048]
              shift-right: [w1045] -> w994
              shift-left: w1004 -> [w1047]
              shift-right: [w1043] -> _
              shift-left: "Adquisicion" ("element") -> [w1044]
              shift-right: [w1042] -> _
              shift-left: _ -> [w1040]
              shift-right: [w1038] -> w993
              shift-left: "" -> [w1037]
              i -> [w1036]
              stop <- w1041 stop-if-true
              n501 = case shown="\"Adquisicion\", Default" w1044 {
                tunnel: w1048 -> [w1056 w1286 w1491 w1653 w1738]
                tunnel: w1047 -> [w1055 w1285 w1490 w1652 w1737]
                tunnel: [w1054 w1286 w1491 w1653 w1738] -> w1046
                tunnel: [w1053 w1285 w1490 w1652 w1737] -> w1045
                tunnel: ["Acel_calib" ("Concept") "Acel_frequency" ("Concept") "Acel_noise" ("Concept") "Acel_result" ("Concept") "Adquisicion" ("Concept")] -> w1043
                tunnel: [sgl[][] [] w1282 w1489 w1651 sgl[][] []] -> w1042
                tunnel: [TRUE w1281 w1488 w1648 FALSE] -> w1035
                tunnel: w1040 -> [_ _ w1479 w1654 w1748]
                tunnel: ["\n" w1279 w1486 w1644 w1736] -> w1039
                frame "Adquisicion", Default {
                  n502 = flat-sequence {
                    tunnel: w1055 -> [w1078]
                    tunnel: w1056 -> [w1079]
                    tunnel: [w1079] -> w1059
                    tunnel: [w1078] -> w1058
                    tunnel: [w1062] -> w1057
                    tunnel: w1059 -> [w1091]
                    tunnel: w1058 -> [w1090]
                    tunnel: w1057 -> [w1087]
                    tunnel: [w1089] -> w1054
                    tunnel: [w1088] -> w1053
                    frame #0 {
                      w1074 = "Calibration" ("element")
                      w1073 = "c"
                      n503 = Format Date/Time String(time format string (%c)="%Y-%m-%d-%H-%M-%S") -> (date/time string=w1065:string)  [unwired: 2 in]
                      n504 = for {
                        N: 1 -> [_]
                        shift-right: [w1080] -> w1060
                        shift-left: _ -> [w1081]
                        n505 = Add(x=w1081, y=0.001) -> (x+y=w1080:dbl)
                      }
                      n506 = Number To Fractional String(number=w1060) -> (F-format string=w1069:string)  [unwired: 3 out]
                      n507 = Search and Replace String(input string=w1069, search string="." ("replace string (\"\")")) -> (result string=w1067:string)  [unwired: 1 in, 8 out]
                      n508 = for {
                        N: 3 -> [_]
                        shift-right: [w1085] -> w1063
                        shift-left: w1067 -> [w1083]
                        n509 = Search and Replace String(input string=w1083, search string="0", offset=4 ("offset (0)")) -> (result string=w1085:string)  [unwired: 1 in, 7 out]
                      }
                      n510 = Concatenate Strings(w1063, "_" ("replace string (\"\")"), w1065) -> (w1062:string)
                      "date/time string 2" <- w1062
                      n511 = Build Array(w1073, w1074, w1062) -> (w1072:string[])
                      n512 = Build Array(w1073, w1074, w1062, "Calibration_LOG.txt" ("element")) -> (w1076:string[])
                      n513 = Array of Strings to Path(0:w1072) -> (2:w1071:path)  [unwired: 1 out]
                      "Folder" <- w1071
                      n514 = Array of Strings to Path(0:w1076) -> (2:→"calibration log":path)  [unwired: 1 out]
                      n515 = Create Folder(path (use dialog)=w1071) -> ()  [unwired: 2 in, 3 out]
                    }
                    frame #1 {
                      n516 = for {
                        N: 11 -> [_]
                        shift-right: [w1110] -> w1089
                        shift-left: w1091 -> [w1120]
                        shift-right: [w1113] -> w1088
                        shift-left: w1090 -> [w1119]
                        tunnel: w1087 -> [w1106]
                        i -> [w1116]
                        n517 = xnode "Invoke Method"("FPGA VI Reference In"=w1120, "error in"=w1119) -> ("FPGA VI Reference Out"=w1118:refnum<k20>, "error out"=w1117:errorcluster)  [unwired: 1 in]
                        n518 = Increment(x=w1116) -> (x+1=w1115:i32)
                        n519 = Number To Decimal String(number=w1115) -> (decimal integer string=w1114:string)  [unwired: 1 in]
                        n520 = flat-sequence {
                          tunnel: w1118 -> [w1131]
                          tunnel: w1117 -> [w1130]
                          tunnel: w1114 -> [w1129]
                          tunnel: [w1131] -> w1112
                          tunnel: [w1130] -> w1111
                          tunnel: [w1124] -> w1107
                          tunnel: w1106 -> [w1124]
                          tunnel: [w1123] -> w1093
                          tunnel: w1112 -> [w1139]
                          tunnel: w1111 -> [w1138]
                          tunnel: [w1139] -> w1109
                          tunnel: [w1138] -> w1108
                          tunnel: w1107 -> [w1136]
                          tunnel: [w1136] -> w1105
                          tunnel: [w1135] -> w1094
                          tunnel: w1093 -> [w1135]
                          tunnel: w1109 -> [w1179]
                          tunnel: w1108 -> [w1178]
                          tunnel: w1105 -> [w1157]
                          tunnel: [w1177] -> w1104
                          tunnel: [w1176] -> w1103
                          tunnel: [w1150] -> w1102
                          tunnel: [w1149] -> w1101
                          tunnel: [w1148] -> w1100
                          tunnel: [w1147] -> w1099
                          tunnel: w1094 -> [w1140]
                          tunnel: w1104 -> [w1206]
                          tunnel: w1103 -> [w1207]
                          tunnel: w1102 -> [w1203]
                          tunnel: w1101 -> [w1202]
                          tunnel: w1100 -> [w1201]
                          tunnel: w1099 -> [w1200]
                          tunnel: [w1205] -> w1098
                          tunnel: [w1197] -> w1097
                          tunnel: [w1194] -> w1096
                          tunnel: [w1193] -> w1095
                          tunnel: [w1272] -> w1113
                          tunnel: [w1273] -> w1110
                          tunnel: w1098 -> [w1275]
                          tunnel: w1097 -> [w1274]
                          tunnel: w1096 -> [w1270]
                          tunnel: w1095 -> [w1269]
                          frame #0 {
                            w1121 = dbl[] [] ("mean")
                            n521 = local read "Report"() -> (w1126:string)
                            n522 = local write "mean"(w1121) -> ()
                            n523 = local write "median"(w1121) -> ()
                            n524 = local write "max"(w1121) -> ()
                            n525 = local write "min"(w1121) -> ()
                            n526 = local write "Value to compare"(w1121) -> ()
                            n527 = Concatenate Strings("\nAcquiring file: ", w1129, "/11\n" ("string"), w1126) -> (w1125:string)
                            n528 = for {
                              N: 1 -> [_]
                              shift-right: [w1132] -> w1123
                              shift-left: _ -> [w1133]
                              n529 = Add(x=w1133, y=0.001) -> (x+y=w1132:dbl)
                            }
                            n530 = local write "Report"(w1125) -> ()
                          }
                          frame #1 {
                            n531 = Wait (ms)(milliseconds to wait=u32 1000) -> ()  [unwired: 1 out]
                          }
                          frame #2 {
                            n532 = local read "Frecuencia de muestreo y módulo CRIO"() -> (w1175:T3)
                            n533 = local read "Frecuencia de muestreo (Hz)"() -> (w1173:dbl)
                            n534 = Number To Fractional String(number=w1140) -> (F-format string=w1154:string)  [unwired: 3 out]
                            n535 = local read "Escaneos de la FIFO por canal"() -> (w1172:u32)
                            n536 = xnode "Read/Write Control"("FPGA VI Reference In"=w1179, "error in"=w1178, "Fotocélula"=TRUE ("Adquirir")) -> ("FPGA VI Reference Out"=w1183:refnum<k20>, "error out"=w1182:errorcluster)
                            n537 = local read "Nº de acelerómetros"() -> (w1170:i32)
                            n538 = local read "Count(mSec)"() -> (w1174:u32)
                            n539 = local read "Nº inductivos"() -> (w1171:i32)
                            n540 = Search and Replace String(input string=w1154, search string="." ("replace string (\"\")")) -> (result string=w1152:string)  [unwired: 1 in, 8 out]
                            n541 = for {
                              N: 3 -> [_]
                              shift-right: [w1191] -> w1155
                              shift-left: w1152 -> [w1189]
                              n542 = Search and Replace String(input string=w1189, search string="0", offset=4 ("offset (0)")) -> (result string=w1191:string)  [unwired: 1 in, 7 out]
                            }
                            n543 = xnode "Read/Write Control"("FPGA VI Reference In"=w1183, "error in"=w1182, "Data Rate"=w1175, "Digital?"=TRUE, "Count(mSec)"=w1174) -> ("FPGA VI Reference Out"=w1185:refnum<k20>, "error out"=w1184:errorcluster)
                            n544 = Format Date/Time String(time format string (%c)="%Y-%m-%d-%H-%M-%S") -> (date/time string=w1156:string)  [unwired: 2 in]
                            n545 = Add(x=w1171, y=w1170) -> (x+y=w1169:i32)
                            n546 = call "DMACalc.vi"("Number of Channels"=w1169, "Number of Samples"=w1172, "Rate (Hz)"=w1173) -> ("Block Size"=w1149:u32, "Time to Acquire Block (ms)"=w1150:i32, "Host Buffer Size"=w1168:u32)  [unwired: 6 in]
                            n547 = xnode "Invoke Method"("FPGA VI Reference In"=w1185, "error in"=w1184, "Requested Depth"=w1168) -> ("FPGA VI Reference Out"=w1187:refnum<k20>, "error out"=w1186:errorcluster)  [unwired: 1 out]
                            n548 = Concatenate Strings(w1155, "_" ("replace string (\"\")"), w1156, ".bin" ("string")) -> (w1163:string)
                            n549 = Build Array("c", "Calibration" ("element"), w1157, w1163) -> (w1162:string[])
                            n550 = xnode "Invoke Method"("FPGA VI Reference In"=w1187, "error in"=w1186) -> ("FPGA VI Reference Out"=w1177:refnum<k20>, "error out"=w1176:errorcluster)
                            n551 = local read "Report"() -> (w1142:string)
                            n552 = Array of Strings to Path(0:w1162) -> (2:w1143:path)  [unwired: 1 out]
                            n553 = Path To String(path=w1143) -> (string=w1146:string)
                            n554 = Get Date/Time In Seconds() -> (seconds since 1Jan1904=→"Inicio pasada 2":timestamp)
                            n555 = Concatenate Strings("\nFile created: ", w1146, "\n", w1142) -> (w1141:string)
                            n556 = Open/Create/Replace File(file path (use dialog)=w1143, operation (0:open)=T5."replace or create", access (0:read/write)=enum16{"read/write", "read-only", "write-only"}."read/write", disable buffering (F)=TRUE) -> (refnum out=w1148:refnum<file>, error out=w1147:errorcluster)  [unwired: 1 in, 2 out]
                            n557 = local write "Report"(w1141) -> ()
                          }
                          frame #3 {
                            n558 = while "Data Acquisition" {
                              tunnel: w1206 -> [w1232]
                              shift-right: [w1239] -> _
                              shift-left: u32 0 ("t") -> [w1235]
                              tunnel: w1203 -> [w1240]
                              tunnel: w1202 -> [w1238]
                              shift-right: [w1241] -> w1197
                              shift-left: w1207 -> [w1231]
                              tunnel: [w1236] -> w1205
                              tunnel: w1201 -> [w1221]
                              tunnel: [w1222] -> w1194
                              shift-right: [w1220] -> w1193
                              shift-left: w1200 -> [w1229]
                              stop <- w1237 stop-if-true
                              # "Detector de presencia"
                              # "Mide el tiempo de paso del tren y con ello se puede calcular\nla velocidad la unidad"
                              n559 = xnode "Invoke Method"("FPGA VI Reference In"=w1232, "error in"=w1231, "Number of Elements"=w1235, "Timeout (ms)"=0) -> ("FPGA VI Reference Out"=w1219:refnum<k20>, "error out"=w1218:errorcluster, "Data"=w1230:fxp<+/-,24,4>[], "Elements Remaining"=w1233:u32)
                              n560 = case "Data Ready" shown="Default" w1235 {
                                tunnel: w1240 -> [w1246 _]
                                tunnel: [w1245 u32 0 ("t")] -> w1239
                                tunnel: w1238 -> [w1247 _]
                                tunnel: w1233 -> [w1244 _]
                                tunnel: w1230 -> [_ w1257]
                                tunnel: w1229 -> [w1243 w1259]
                                tunnel: [w1243 w1258] -> w1220
                                tunnel: w1221 -> [w1242 w1256]
                                tunnel: [w1242 w1255] -> w1222
                                frame 0 {
                                n561 = Greater Or Equal?(x=w1244, y=w1247) -> (x >= y?=w1248:bool)
                                n562 = case shown="False" w1248 {
                                tunnel: [u32 0 ("Block Size") w1252] -> w1245
                                tunnel: [w1251 0 ("t")] -> w1249
                                tunnel: w1246 -> [w1251 _]
                                tunnel: w1247 -> [_ w1252]
                                frame False {
                                }
                                frame True {
                                }
                                }
                                n563 = call "WaitMinTimeBetweenCall.vi"("Minimum ms between calls"=w1249) -> ()  [unwired: 2 in]
                                }
                                frame Default {
                                n564 = To Single Precision Float(number=w1257) -> (single precision float=w1254:sgl[])
                                n565 = Write to Binary File(file (use dialog)=w1256, data=w1254, error in=w1259, 5:FALSE ("prepend array or string size? (T)"), 9:T6."little-endian" ("byte order (0:big-endian, network order)")) -> (refnum out=w1255:refnum<file>, error out=w1258:errorcluster)  [unwired: 2 out]
                                }
                              }
                              n566 = local read "Inicio pasada 2"() -> (w1210:timestamp)
                              n567 = Get Date/Time In Seconds() -> (seconds since 1Jan1904=w1211:timestamp)
                              n568 = xnode ("CheckLate")("FPGA VI Reference In"=w1219, "error in"=w1218) -> ("FPGA VI Reference Out"=w1213:refnum<k20>, "error out"=w1227:errorcluster, "Buffer Underflow"=w1208:bool, "Buffer Overflow"=w1209:bool)
                              n569 = To Double Precision Float(number=w1211) -> (double precision float=w1216:dbl)
                              n570 = To Double Precision Float(number=w1210) -> (double precision float=w1217:dbl)
                              n571 = Subtract(x=w1216, y=w1217) -> (x-y=w1224:dbl)
                              "Acquiring time" <- w1224
                              n572 = local write "Buffer Overflow"(w1209) -> ()
                              n573 = local write "Buffer Underflow"(w1208) -> ()
                              n574 = Greater?(x=w1224, y=1.0 ("Tiempo de adquisición")) -> (0:w1215:bool)
                              n575 = call "ErrorOverFlow.vi"("Buffer Overflow"=w1209) -> ("error out"=w1225:errorcluster)
                              n576 = call "ErrorUnderFlow.vi"("Buffer Overflow"=w1208) -> ("error out"=w1226:errorcluster)
                              n577 = Merge Errors(w1227, w1226, w1225) -> (w1214:errorcluster)
                              n578 = Unbundle By Name(w1220) -> ("status"=w1223:bool)
                              n579 = Unbundle By Name(w1214) -> ("status"=w1228:bool)
                              n580 = Compound Arithmetic op=OR(w1228, w1215, w1223) -> (w1237:bool)
                              n581 = case "Flush" shown="True" w1237 {
                                tunnel: w1213 -> [w1263 w1268]
                                tunnel: w1214 -> [w1264 w1267]
                                tunnel: [w1264 w1266] -> w1241
                                tunnel: [w1263 w1265] -> w1236
                                frame False {
                                }
                                frame True {
                                n582 = xnode "Invoke Method"("FPGA VI Reference In"=w1268, "error in"=w1267) -> ("FPGA VI Reference Out"=w1265:refnum<k20>, "error out"=w1266:errorcluster)
                                }
                              }
                            }
                            n583 = call "Reporting_error.vi"("error out 2"=w1197, "Concept"="FPGA ") -> ("Reporting"=w1199:string)  [unwired: 1 in]
                            n584 = local read "Report"() -> (w1196:string)
                            n585 = Concatenate Strings(w1199, w1196) -> (w1198:string)
                            n586 = local write "Report"(w1198) -> ()
                          }
                          frame #4 {
                            n587 = xnode "Read/Write Control"("FPGA VI Reference In"=w1275, "error in"=w1274, "Stop"=TRUE) -> ("FPGA VI Reference Out"=w1276:refnum<k20>, "error out"=w1277:errorcluster)
                            n588 = Close File(refnum=w1270, error in=w1269) -> ()  [unwired: 2 out]
                            n589 = xnode "Invoke Method"("FPGA VI Reference In"=w1276, "error in"=w1277) -> ("FPGA VI Reference Out"=w1273:refnum<k20>, "error out"=w1272:errorcluster)
                          }
                        }
                      }
                    }
                  }
                }
                frame "Acel_calib" {
                  n590 = local read "Folder"() -> (w1288:path)
                  n591 = local read "Frecuencia de muestreo (Hz)"() -> (w1294:dbl)
                  n592 = local read "Nº de acelerómetros"() -> (w1289:i32)
                  n593 = local read "Nº inductivos"() -> (w1290:i32)
                  n594 = local read "Pattern frequency (Hz)"() -> (w1295:dbl)
                  n595 = call <vilib>:"Recursive File List.vi"("Folder Path"=w1288) -> ("All Files in Dir"=w1293:path[])  [unwired: 6 in, 4 out]
                  n596 = Array Size(array=w1293) -> (size(s)=→"Nº meas":i32)
                  n597 = Add(x=w1290, y=w1289) -> (x+y=w1292:i32)
                  n598 = flat-sequence {
                    tunnel: w1293 -> [w1305]
                    tunnel: [w1305] -> w1301
                    tunnel: [w1304] -> w1300
                    tunnel: w1292 -> [w1304]
                    tunnel: [w1303] -> w1299
                    tunnel: w1294 -> [w1303]
                    tunnel: [w1302] -> w1298
                    tunnel: w1295 -> [w1302]
                    tunnel: [w1312] -> w1297
                    tunnel: [w1311] -> w1296
                    tunnel: w1301 -> [w1313]
                    tunnel: w1300 -> [w1310]
                    tunnel: w1299 -> [w1309]
                    tunnel: w1298 -> [w1308]
                    tunnel: [w1307] -> w1278
                    tunnel: w1297 -> [w1425]
                    tunnel: w1296 -> [w1414]
                    tunnel: [w1406] -> w1282
                    tunnel: [TRUE] -> w1281
                    tunnel: [w1440] -> w1279
                    tunnel: [w1415] -> w1280
                    tunnel: w1278 -> [w1410]
                    frame #0 {
                      "Valid\nindex" <- i32[] []
                    }
                    frame #1 {
                      n599 = for {
                        tunnel: w1313 -> [w1335] mode=indexing
                        tunnel: [w1325] -> w1312 mode=indexing
                        tunnel: [w1315] -> w1311 mode=indexing
                        tunnel: w1310 -> [w1323]
                        tunnel: w1309 -> [w1322]
                        tunnel: w1308 -> [w1321]
                        tunnel: [w1314] -> w1307 mode=indexing
                        n600 = Read from Binary File(5:sgl 1.25, 9:T6."little-endian" ("byte order (0:big-endian, network order)"), 10:-1 ("count (1)"), 11:w1335) -> (2:w1336:sgl[])  [unwired: 1 in, 4 out]
                        n601 = case shown="10" w1323 {
                          tunnel: [w1353 w1366 w1376] -> w1315
                          tunnel: w1336 -> [w1354 w1364 w1377]
                          frame 9, Default {
                            n602 = Decimate 1D Array(w1354) -> (w1355:sgl[], w1363:sgl[], w1362:sgl[], w1358:sgl[], w1357:sgl[], w1359:sgl[], w1360:sgl[], w1361:sgl[], w1356:sgl[])
                            n603 = Build Array(w1355, w1363, w1362, w1358, w1357, w1359, w1360, w1361, w1356) -> (w1353:sgl[][])
                          }
                          frame 10 {
                            n604 = Decimate 1D Array(w1364) -> (w1365:sgl[], w1375:sgl[], w1374:sgl[], w1370:sgl[], w1369:sgl[], w1371:sgl[], w1372:sgl[], w1373:sgl[], w1368:sgl[], w1367:sgl[])
                            n605 = Build Array(w1365, w1375, w1374, w1370, w1369, w1371, w1372, w1373, w1368, w1367) -> (w1366:sgl[][])
                          }
                          frame 5 {
                            n606 = Decimate 1D Array(w1377) -> (w1378:sgl[], w1382:sgl[], w1381:sgl[], w1380:sgl[], w1379:sgl[])
                            n607 = Build Array(w1378, w1382, w1381, w1380, w1379) -> (w1376:sgl[][])
                          }
                        }
                        n608 = for {
                          tunnel: w1315 -> [w1385] mode=indexing
                          tunnel: [w1388] -> w1332 mode=indexing
                          tunnel: w1322 -> [w1387]
                          tunnel: w1321 -> [w1386]
                          n609 = call-poly <vilib>:"Basic Averaged DC-RMS.vi"("signal in"=w1385) -> ("DC value"=w1398:dbl)  [unwired: 7 in, 3 out]
                          n610 = Array Size(array=w1385) -> (size(s)=→"size(s) 3":i32)
                          n611 = Subtract(x=w1385, y=w1398) -> (x-y=w1394:dbl[])
                          n612 = Divide(x=w1387, y=w1386) -> (x/y=w1395:dbl)
                          n613 = Array Size(array=w1394) -> (size(s)=w1396:i32)
                          n614 = Subtract(x=w1396, y=w1395) -> (x-y=w1397:dbl)
                          n615 = for {
                            N: w1397 -> [_]
                            tunnel: w1395 -> [w1400]
                            tunnel: [w1403] -> w1383 mode=indexing
                            tunnel: w1394 -> [w1402]
                            i -> [w1401]
                            n616 = Array Subset(array=w1402, index=w1401, length=w1400) -> (w1399:dbl[])
                            n617 = call-poly <vilib>:"RMS.vi"("X"=w1399) -> ("rms value"=w1403:dbl)  [unwired: 1 out]
                          }
                          n618 = Greater?(x=w1383, y=0.004 ("threshold y")) -> (0:w1392:bool[])
                          n619 = Search 1D Array(1D array=w1392, element=TRUE) -> (index of element=w1390:i32)  [unwired: 1 in]
                          n620 = Not Equal?(x=w1390, y=-1) -> (x != y?=w1388:bool)
                        }
                        n621 = Array Size(array=w1315) -> (size(s)=→"size(s)":i32[])
                        n622 = while {
                          tunnel: w1332 -> [w1352]
                          shift-right: [w1344] -> _
                          shift-left: 0 ("index of element") -> [w1349]
                          shift-right: [w1345] -> w1324
                          shift-left: 0 ("index of element") -> [w1346]
                          tunnel: [w1343] -> w1320 mode=indexing
                          i -> [w1347]
                          stop <- w1350 stop-if-true
                          n623 = Add(x=w1346, y=w1347) -> (x+y=w1345:i32)
                          n624 = Search 1D Array(1D array=w1352, element=TRUE, start index (0)=w1349) -> (index of element=w1343:i32)
                          n625 = Equal?(x=w1343, y=-1) -> (x = y?=w1350:bool)
                          n626 = Increment(x=w1343) -> (x+1=w1344:i32)
                        }
                        n627 = Delete From Array(array=w1320, length=1) -> (array with subset deleted=w1319:i32[])  [unwired: 1 in, 1 out]
                        n628 = Array Size(array=w1319) -> (size(s)=w1328:i32)
                        n629 = Equal?(x=w1324, y=1) -> (x = y?=w1327:bool)
                        n630 = Equal?(x=w1328, y=1) -> (x = y?=w1326:bool)
                        n631 = And(x=w1326, y=w1327) -> (x .and. y?=w1325:bool)
                        n632 = case shown="True" w1325 {
                          tunnel: w1319 -> [_ w1342]
                          frame False {
                          }
                          frame True {
                            n633 = local read "Valid\nindex"() -> (w1340:i32[])
                            n634 = Insert Into Array(array=w1340, new element=w1342) -> (w1341:i32[])  [unwired: 1 in]
                            n635 = local write "Valid\nindex"(w1341) -> ()
                          }
                        }
                        n636 = Array Size(array=w1315) -> (size(s)=w1317:i32[])
                        n637 = Index Array(array=w1317, index=1) -> (element=w1314:i32)
                      }
                    }
                    frame #2 {
                      w1424 = 0 ("index of element")
                      (unwired) 0 ("index of element")
                      n638 = local read "Valid\nindex"() -> (w1430:i32[])
                      n639 = Array Max & Min(array=w1410) -> (min value=w1407:i32)  [unwired: 3 out]
                      n640 = Sort 1D Array(array=w1430) -> (sorted array=w1426:i32[])
                      "sorted array" <- w1426
                      n641 = Decrement(x="Accelerometer") -> (x-1=w1405:i32)
                      n642 = for {
                        tunnel: w1426 -> [w1461] mode=indexing
                        shift-right: [w1461] -> _
                        shift-left: -1 ("y") -> [w1462]
                        tunnel: [w1461] -> w1435 mode=indexing if=w1460
                        shift-right: [w1457] -> _
                        shift-left: 0 ("y") -> [w1458]
                        tunnel: [w1457] -> w1433 mode=indexing
                        n643 = Not Equal?(x=w1461, y=w1462) -> (x != y?=w1460:bool)
                        n644 = Increment(x=w1458) -> (x+1=w1459:i32)
                        n645 = Select(t=1 ("y"), s=w1460, f=w1459) -> (s? t:f=w1457:i32)
                      }
                      "Array" <- w1435
                      "Array 3" <- w1433
                      n646 = Delete From Array(array=w1414, index (dim 1)=w1405) -> (deleted portion=w1408:sgl[][])  [unwired: 3 in, 1 out]
                      n647 = for {
                        tunnel: w1425 -> [w1467] mode=indexing
                        shift-right: [w1466] -> _
                        shift-left: w1414 -> [w1468]
                        shift-right: [w1463] -> _
                        shift-left: 0 ("index of element") -> [w1464]
                        i -> [w1465]
                        n648 = case shown="False" w1467 {
                          tunnel: w1468 -> [w1474 w1476]
                          tunnel: [w1473 w1476] -> w1466
                          tunnel: w1465 -> [w1472 _]
                          tunnel: w1464 -> [w1469 w1475]
                          tunnel: [w1470 w1475] -> w1463
                          frame False {
                            n649 = Subtract(x=w1472, y=w1469) -> (x-y=w1471:i32)
                            n650 = Delete From Array(array=w1474, index (dim 0)=w1471) -> (array with subset deleted=w1473:sgl[][][])  [unwired: 3 in, 1 out]
                            n651 = Increment(x=w1469) -> (x+1=w1470:i32)
                          }
                          frame True {
                          }
                        }
                      }
                      n652 = Array Subset(array=w1408, index (col)=0 ("index"), length (col)=w1407) -> (w1406:sgl[][])  [unwired: 2 in]
                      n653 = Array Max & Min(array=w1433) -> (max value=→"max value":i32, max index (indices)=w1431:i32)  [unwired: 2 out]
                      "max index(es)" <- w1431
                      n654 = Index Array(array=w1426, index=w1431) -> (element=w1415:i32)
                      "element" <- w1415
                      n655 = local read "Frecuencia de muestreo (Hz)"() -> (w1413:dbl)
                      n656 = Equal?(x=w1430, y=w1415) -> (x = y?=w1428:bool[])
                      n657 = Boolean To (0,1)(Boolean=w1428) -> (0, 1=w1427:i16[])
                      n658 = Add Array Elements(numeric array=w1427) -> (sum=w1419:i16)
                      n659 = Equal?(x=w1415, y=w1424) -> (x = y?=w1422:bool)
                      n660 = Equal?(x=w1424, y=w1419) -> (x = y?=w1421:bool)
                      n661 = Increment(x=w1415) -> (x+1=w1429:i32)
                      n662 = local read "Nº meas"() -> (w1441:i32)
                      n663 = Not And(1:w1421, 2:w1422) -> (0:w1420:bool)
                      n664 = for {
                        tunnel: w1406 -> [w1455] mode=indexing
                        tunnel: w1413 -> [w1453]
                        tunnel: [w1452] -> w1412 mode=indexing
                        n665 = Reciprocal(x=w1453) -> (1/x=w1454:dbl)
                        n666 = Bundle By Name("Y"=w1455, "dt"=w1454) -> (w1452:waveform(sgl))  [unwired: 1 in]
                      }
                      n667 = Number To Decimal String(number=w1429) -> (decimal integer string=w1417:string)  [unwired: 1 in]
                      n668 = Select(t=w1417, s=w1420, f=" NONE ") -> (s? t:f=w1418:string)
                      n669 = Number To Decimal String(number=w1419) -> (decimal integer string=w1447:string)  [unwired: 1 in]
                      n670 = Number To Decimal String(number=w1441) -> (decimal integer string=w1445:string)  [unwired: 1 in]
                      n671 = Divide(x=w1419, y=w1441) -> (x/y=w1443:dbl)
                      n672 = for {
                        tunnel: w1412 -> [w1451] mode=indexing
                        tunnel: [w1448] -> w1411 mode=concatenating
                        n673 = call "Convert to Dynamic Data"("Waveform"=w1451) -> ("Dynamic Data Type"=w1450:dynamicdata)  [unwired: 3 in]
                        n674 = call "Tone Measurements"("Signals"=w1450) -> ("Frequency"=w1449:dynamicdata)  [unwired: 9 in, 1 out]
                        n675 = call "Convert from Dynamic Data"("Dynamic Data Type"=w1449) -> ("Array"=w1448:dbl[])  [unwired: 3 in]
                      }
                      "Frequency" <- w1411
                      n676 = Greater?(x=w1443, y=0.6) -> ()  [unwired: 1 out]
                      n677 = Concatenate Strings("\nACCELEROMETER DETECTOR:\n\nAccelerometer detected: ", w1418, " \nAccelerometer detected in  ", w1447, " of ", w1445, " measurements\n------------------------------------------------------------------------------------------------------------------------------------------------") -> (w1440:string)
                    }
                  }
                  n678 = local read "Report"() -> (w1283:string)
                  n679 = Concatenate Strings(w1279, w1283) -> (w1284:string)
                  n680 = local write "Report"(w1284) -> ()
                  "Accel.detected" <- w1280
                }
                frame "Acel_frequency" {
                  n681 = local read "Low cutoff freq"() -> (w1481:dbl)
                  n682 = local read "Frequency"() -> (w1482:dbl[])
                  n683 = local read "Frecuencia de muestreo (Hz)"() -> (w1484:dbl)
                  n684 = for {
                    tunnel: w1479 -> [w1515] mode=indexing
                    tunnel: w1484 -> [w1513]
                    tunnel: [w1512] -> w1483 mode=indexing
                    n685 = Reciprocal(x=w1513) -> (1/x=w1514:dbl)
                    n686 = Bundle By Name("Y"=w1515, "dt"=w1514) -> (w1512:waveform(sgl))  [unwired: 1 in]
                  }
                  "Waveform Graph" <- w1483
                  n687 = local read "Pattern frequency (Hz)"() -> (w1485:dbl)
                  n688 = Less?(x=w1482, y=w1481) -> (x < y?=w1477:bool[])
                  n689 = for {
                    tunnel: w1477 -> [w1502] mode=indexing
                    shift-right: [w1501] -> w1478
                    shift-left: w1479 -> [w1503]
                    shift-right: [w1498] -> _
                    shift-left: 0 ("index of element") -> [w1499]
                    i -> [w1500]
                    n690 = case shown="False" w1502 {
                      tunnel: w1503 -> [w1509 w1511]
                      tunnel: [w1508 w1511] -> w1501
                      tunnel: w1500 -> [w1507 _]
                      tunnel: w1499 -> [w1504 w1510]
                      tunnel: [w1505 w1510] -> w1498
                      frame False {
                        n691 = Subtract(x=w1507, y=w1504) -> (x-y=w1506:i32)
                        n692 = Delete From Array(array=w1509, index (row)=w1506) -> (array with subset deleted=w1508:sgl[][])  [unwired: 2 in, 1 out]
                        n693 = Increment(x=w1504) -> (x+1=w1505:i32)
                      }
                      frame True {
                      }
                    }
                  }
                  n694 = flat-sequence {
                    tunnel: w1478 -> [w1522]
                    tunnel: w1484 -> [w1519]
                    tunnel: w1485 -> [w1516]
                    tunnel: [w1524] -> w1497
                    tunnel: [w1518] -> w1496
                    tunnel: [w1517] -> w1495
                    tunnel: [w1516] -> w1494
                    tunnel: w1497 -> [w1601]
                    tunnel: w1496 -> [w1583]
                    tunnel: w1495 -> [w1600]
                    tunnel: w1494 -> [w1599]
                    tunnel: [w1601] -> w1489
                    tunnel: [w1585] -> w1486
                    tunnel: [w1584] -> w1488
                    tunnel: [w1583] -> _
                    frame #0 {
                      n695 = for {
                        tunnel: w1522 -> [w1574] mode=indexing
                        tunnel: w1519 -> [w1573]
                        tunnel: w1516 -> [w1569]
                        tunnel: [w1550] -> w1518 mode=indexing
                        tunnel: [w1544] -> w1517 mode=indexing
                        n696 = Reciprocal(x=w1573) -> (1/x=w1575:dbl)
                        n697 = Bundle By Name("Y"=w1574, "dt"=w1575) -> (w1572:waveform(sgl))  [unwired: 1 in]
                        n698 = call-poly <vilib>:"FFT Spectrum (Mag-Phase).vi"("time signal"=w1572) -> ("magnitude"=w1571:cluster{"f0":dbl, "df":dbl, "magnitude":dbl[]})  [unwired: 6 in, 4 out]
                        n699 = Unbundle By Name(w1571) -> ("magnitude"=w1563:dbl[], "df"=w1545:dbl)
                        n700 = Multiply(x=1.03, y=w1569) -> (x*y=w1566:dbl)
                        n701 = Multiply(x=w1569, y=0.97 ("x")) -> (x*y=w1567:dbl)
                        n702 = Divide(x=w1567, y=w1545) -> (x/y=w1564:dbl)
                        n703 = Divide(x=w1566, y=w1545) -> (x/y=w1561:dbl)
                        n704 = Array Max & Min(array=w1563) -> (max value=w1556:dbl, max index (indices)=w1546:i32)  [unwired: 2 out]
                        n705 = Array Size(array=w1563) -> (size(s)=w1562:i32)
                        n706 = Multiply(x=w1546, y=w1545) -> (x*y=w1544:dbl)
                        n707 = Subtract(x=w1562, y=w1561) -> (x-y=w1560:dbl)
                        n708 = In Range and Coerce(upper limit=w1566, x=w1544, lower limit=w1567) -> (In Range?=w1549:bool)  [unwired: 1 out]
                        n709 = Array Subset(array=w1563, index=w1561, length=w1560) -> (w1559:dbl[])
                        n710 = Array Subset(array=w1563, index=0, length=w1564) -> (w1558:dbl[])
                        n711 = Array Max & Min(array=w1559) -> (max value=w1557:dbl)  [unwired: 3 out]
                        n712 = Array Max & Min(array=w1558) -> (max value=w1555:dbl)  [unwired: 3 out]
                        n713 = Divide(x=w1556, y=w1555) -> (x/y=w1553:dbl)
                        n714 = Divide(x=w1556, y=w1557) -> (x/y=w1554:dbl)
                        n715 = Greater?(x=w1554, y=3.0) -> (0:w1548:bool)
                        n716 = Greater?(x=w1553, y=3.0) -> (0:w1547:bool)
                        n717 = Compound Arithmetic op=AND(w1549, w1548, w1547) -> (w1550:bool)
                      }
                      n718 = for {
                        shift-right: [w1531] -> w1524
                        shift-left: w1522 -> [w1532]
                        tunnel: w1518 -> [w1530] mode=indexing
                        shift-right: [w1527] -> _
                        shift-left: 0 ("index of element") -> [w1528]
                        shift-right: [w1525] -> w1521
                        shift-left: w1517 -> [w1526]
                        i -> [w1529]
                        n719 = case shown="True" w1530 {
                          tunnel: w1532 -> [w1540 w1543]
                          tunnel: [w1539 w1543] -> w1531
                          tunnel: w1529 -> [w1538 _]
                          tunnel: w1528 -> [w1537 w1542]
                          tunnel: [w1536 w1542] -> w1527
                          tunnel: w1526 -> [w1535 w1541]
                          tunnel: [w1533 w1541] -> w1525
                          frame False {
                            n720 = Subtract(x=w1538, y=w1537) -> (x-y=w1534:i32)
                            n721 = Delete From Array(array=w1540, index (row)=w1534) -> (array with subset deleted=w1539:sgl[][])  [unwired: 2 in, 1 out]
                            n722 = Increment(x=w1537) -> (x+1=w1536:i32)
                            n723 = Delete From Array(array=w1535, index=w1534) -> (array with subset deleted=w1533:dbl[])  [unwired: 1 in, 1 out]
                          }
                          frame True {
                          }
                        }
                      }
                      n724 = call <vilib>:"Std Deviation and Variance.vi"("X"=w1521) -> ("mean"=→"Mean\nfrequency":dbl)  [unwired: 1 in, 2 out]
                    }
                    frame #1 {
                      w1580 = "\r"
                      n725 = for {
                        tunnel: w1583 -> [w1609] mode=indexing
                        tunnel: w1600 -> [w1628] mode=indexing
                        tunnel: w1599 -> [w1627]
                        tunnel: [w1610] -> w1597 mode=indexing
                        shift-right: [w1604] -> w1595
                        shift-left: 0 -> [w1605]
                        i -> [w1630]
                        n726 = Increment(x=w1630) -> (x+1=w1629:i32)
                        n727 = Select(t=1, s=w1609, f=0) -> (s? t:f=w1606:i32)
                        n728 = Divide(x=w1628, y=w1627) -> (x/y=w1625:dbl)
                        n729 = Select(t="TRUE", s=w1609, f="FALSE") -> (s? t:f=w1619:string)
                        n730 = Number To Decimal String(number=w1629) -> (decimal integer string=w1622:string)  [unwired: 1 in]
                        n731 = Number To Fractional String(number=w1628, precision (6)=i16 2) -> (F-format string=w1616:string)  [unwired: 2 in]
                        n732 = Add(x=w1606, y=w1605) -> (x+y=w1604:i32)
                        n733 = Greater Than 0?(x=w1625) -> (x > 0?=w1626:bool)
                        n734 = case shown="True" w1626 {
                          tunnel: w1625 -> [w1638 w1640]
                          tunnel: [w1634 w1642] -> w1624
                          tunnel: ["-" " "] -> w1614
                          frame False {
                            n735 = Subtract(x=1.0, y=w1638) -> (x-y=w1636:dbl)
                            n736 = Multiply(x=100.0, y=w1636) -> (x*y=w1634:dbl)
                          }
                          frame True {
                            n737 = Decrement(x=w1640) -> (x-1=w1641:dbl)
                            n738 = Multiply(x=100.0, y=w1641) -> (x*y=w1642:dbl)
                          }
                        }
                        n739 = Number To Fractional String(number=w1624, precision (6)=i16 2) -> (F-format string=w1613:string)  [unwired: 2 in]
                        n740 = Concatenate Strings("\n\nMeasurement: ", w1622, "\r", "Frequency valid: ", w1619, "\r", "Frequency: ", w1616, ", ", w1614, w1613, " % of error in frequency", "\r") -> (w1610:string)
                      }
                      n741 = Array Size(array=w1583) -> (size(s)=w1594:i32)
                      n742 = Number To Decimal String(number=w1594) -> (decimal integer string=w1589:string)  [unwired: 1 in]
                      n743 = Number To Decimal String(number=w1595) -> (decimal integer string=w1581:string)  [unwired: 1 in]
                      n744 = Divide(x=w1595, y=w1594) -> (x/y=w1578:dbl)
                      n745 = Greater?(x=w1578, y=0.8) -> (0:w1584:bool)
                      n746 = Multiply(x=100.0, y=w1578) -> (x*y=w1577:dbl)
                      n747 = Number To Fractional String(number=w1577, precision (6)=i16 2) -> (F-format string=w1588:string)  [unwired: 2 in]
                      n748 = Select(t="OK\n------------------------------------------------------------------------", s=w1584, f="FAIL (REPEAT ACEL CALIBRATION)\n------------------------------------------------------------------------") -> (s? t:f=w1586:string)
                      n749 = Concatenate Strings("FREQUENCY TEST:\n \n- MEASUREMENT OK IF +/- 5% FREQ PATTERN\n\n- FREQUENCY ANALYSYS MORE THAN 80% OF THE MEASUREMENTS INSIDE OF THE RANGE\n", w1597, w1580, w1580, w1581, " measurements OK of ", w1589, " , ", w1588, " %\n\nFREQUENCY ANALYSIS: ", w1586) -> (w1585:string)
                    }
                  }
                  n750 = local read "Report"() -> (w1493:string)
                  n751 = Concatenate Strings(w1486, w1493) -> (w1492:string)
                  n752 = local write "Report"(w1492) -> ()
                }
                frame "Acel_noise" {
                  n753 = local read "Frecuencia de muestreo (Hz)"() -> (w1647:dbl)
                  n754 = local read "Pattern frequency (Hz)"() -> (w1646:dbl)
                  n755 = flat-sequence {
                    tunnel: w1654 -> [w1665]
                    tunnel: [w1681] -> w1651
                    tunnel: w1647 -> [w1680]
                    tunnel: w1646 -> [w1679]
                    tunnel: [w1668] -> w1644
                    tunnel: [w1667] -> w1648
                    frame #0 {
                      n756 = for {
                        tunnel: w1665 -> [w1729] mode=indexing
                        tunnel: [w1722] -> w1685 mode=indexing
                        tunnel: w1680 -> [w1717]
                        tunnel: w1679 -> [w1718]
                        n757 = call-poly <vilib>:"Basic Averaged DC-RMS.vi"("signal in"=w1729) -> ("DC value"=w1730:dbl)  [unwired: 7 in, 3 out]
                        n758 = Subtract(x=w1729, y=w1730) -> (x-y=w1719:dbl[])
                        n759 = Divide(x=w1717, y=w1718) -> (x/y=w1726:dbl)
                        n760 = Array Size(array=w1719) -> (size(s)=w1727:i32)
                        n761 = Subtract(x=w1727, y=w1726) -> (x-y=w1728:dbl)
                        n762 = for {
                          N: w1728 -> [_]
                          tunnel: w1726 -> [w1732]
                          tunnel: [w1735] -> w1720 mode=indexing
                          tunnel: w1719 -> [w1734]
                          i -> [w1733]
                          n763 = Array Subset(array=w1734, index=w1733, length=w1732) -> (w1731:dbl[])
                          n764 = call-poly <vilib>:"RMS.vi"("X"=w1731) -> ("rms value"=w1735:dbl)  [unwired: 1 out]
                        }
                        n765 = Array Max & Min(array=w1720) -> (max value=w1724:dbl, min value=w1723:dbl)  [unwired: 2 out]
                        n766 = call <vilib>:"Std Deviation and Variance.vi"("X"=w1720) -> ("mean"=w1721:dbl)  [unwired: 1 in, 2 out]
                        n767 = call <vilib>:"Median.vi"("X"=w1720) -> ("median"=w1725:dbl)  [unwired: 1 out]
                        n768 = Build Array(w1721, w1725, w1724, w1723) -> (w1722:dbl[])
                      }
                      n769 = Multiply(x=w1685, y=1000 ("median")) -> (x*y=w1664:dbl[][])
                      n770 = Index Array(array=w1664, index (col) #1=0 ("disabled index (col)"), index (col) #2=1 ("index (col)"), index (col) #3=2 ("index (col)"), index (col) #4=3 ("index (col)")) -> (element #1=→"mean":dbl[], element #2=→"median":dbl[], element #3=→"max":dbl[], element #4=→"min":dbl[])  [unwired: 4 in]
                      n771 = for {
                        tunnel: w1664 -> [w1712] mode=indexing
                        tunnel: [w1709] -> w1666 mode=indexing
                        tunnel: [w1707] -> w1655 mode=indexing
                        (unwired) 0.2 ("x")
                        n772 = local read "noise_range"() -> (w1708:dbl)
                        n773 = call <vilib>:"Median.vi"("X"=w1712) -> ("median"=w1707:dbl)  [unwired: 1 out]
                        n774 = Subtract(x=w1707, y=w1708) -> (x-y=w1710:dbl)
                        n775 = Add(x=w1708, y=w1707) -> (x+y=w1711:dbl)
                        n776 = for {
                          tunnel: w1712 -> [w1716] mode=indexing
                          tunnel: w1711 -> [w1715]
                          tunnel: w1710 -> [w1714]
                          tunnel: [w1713] -> w1709 mode=indexing
                          n777 = In Range and Coerce(upper limit=w1715, x=w1716, lower limit=w1714) -> (In Range?=w1713:bool)  [unwired: 1 out]
                        }
                      }
                      "Value to compare" <- w1655
                      n778 = for {
                        tunnel: w1666 -> [w1706] mode=indexing
                        tunnel: [w1705] -> w1682 mode=indexing
                        n779 = And Array Elements(Boolean array=w1706) -> (logical AND=w1705:bool)
                      }
                      n780 = for {
                        shift-right: [w1692] -> w1681
                        shift-left: w1665 -> [w1693]
                        tunnel: w1682 -> [w1691] mode=indexing
                        shift-right: [w1688] -> w1678
                        shift-left: 0 ("index of element") -> [w1689]
                        shift-right: [w1686] -> w1673
                        shift-left: 0 ("index of element") -> [w1687]
                        i -> [w1690]
                        n781 = case shown="False" w1691 {
                          tunnel: w1693 -> [w1700 w1704]
                          tunnel: [w1699 w1704] -> w1692
                          tunnel: w1690 -> [w1698 _]
                          tunnel: w1689 -> [w1697 w1703]
                          tunnel: [w1696 w1703] -> w1688
                          tunnel: w1687 -> [w1694 w1702]
                          tunnel: [w1694 w1701] -> w1686
                          frame False {
                            n782 = Subtract(x=w1698, y=w1697) -> (x-y=w1695:i32)
                            n783 = Delete From Array(array=w1700, index (row)=w1695) -> (array with subset deleted=w1699:sgl[][])  [unwired: 2 in, 1 out]
                            n784 = Increment(x=w1697) -> (x+1=w1696:i32)
                          }
                          frame True {
                            n785 = Increment(x=w1702) -> (x+1=w1701:i32)
                          }
                        }
                      }
                      n786 = Number To Decimal String(number=w1678) -> (decimal integer string=w1676:string)  [unwired: 1 in]
                      n787 = Greater?(x=w1673, y=3) -> (0:w1667:bool)
                      n788 = Select(t="------------------------------------------------------------------------", s=w1667, f="There are not enough correct measurements to calibrate\n\nREPEAT THE ACCELEROMETER CALIBRATION\n------------------------------------------------------------------------") -> (s? t:f=w1669:string)
                      n789 = Concatenate Strings("SIGNAL NOISE ANALYSIS:\n\nFiles erasing by  noise: ", w1676, "\r", w1669) -> (w1668:string)
                    }
                  }
                  n790 = local read "Report"() -> (w1649:string)
                  n791 = Concatenate Strings(w1644, w1649) -> (w1650:string)
                  n792 = local write "Report"(w1650) -> ()
                }
                frame "Acel_result" {
                  n793 = local read "Frecuencia de muestreo (Hz)"() -> (w1747:dbl)
                  n794 = local read "Pattern frequency (Hz)"() -> (w1746:dbl)
                  n795 = local read "Pattern amplitude (g)"() -> (w1745:dbl)
                  n796 = flat-sequence {
                    tunnel: w1748 -> [w1766]
                    tunnel: w1747 -> [w1764]
                    tunnel: w1746 -> [w1763]
                    tunnel: w1745 -> [w1762]
                    tunnel: [w1761] -> w1741
                    tunnel: [w1752] -> _
                    tunnel: [w1751] -> w1736
                    frame #0 {
                      n797 = for {
                        tunnel: w1766 -> [w1780] mode=indexing
                        tunnel: w1764 -> [w1776]
                        tunnel: w1763 -> [w1773]
                        tunnel: [w1774] -> w1771 mode=indexing
                        n798 = call-poly <vilib>:"Basic Averaged DC-RMS.vi"("signal in"=w1780) -> ("DC value"=w1781:dbl)  [unwired: 7 in, 3 out]
                        n799 = Subtract(x=w1780, y=w1781) -> (x-y=w1772:dbl[])
                        n800 = Divide(x=w1776, y=w1773) -> (x/y=w1777:dbl)
                        n801 = Array Size(array=w1772) -> (size(s)=w1778:i32)
                        n802 = Subtract(x=w1778, y=w1777) -> (x-y=w1779:dbl)
                        n803 = for {
                          N: w1779 -> [_]
                          tunnel: w1777 -> [w1783]
                          tunnel: [w1786] -> w1775 mode=indexing
                          tunnel: w1772 -> [w1785]
                          i -> [w1784]
                          n804 = Array Subset(array=w1785, index=w1784, length=w1783) -> (w1782:dbl[])
                          n805 = call-poly <vilib>:"RMS.vi"("X"=w1782) -> ("rms value"=w1786:dbl)  [unwired: 1 out]
                        }
                        n806 = call <vilib>:"Std Deviation and Variance.vi"("X"=w1775) -> ("mean"=w1774:dbl)  [unwired: 1 in, 2 out]
                      }
                      n807 = call <vilib>:"Std Deviation and Variance.vi"("X"=w1771) -> ("mean"=w1770:dbl)  [unwired: 1 in, 2 out]
                      n808 = Divide(x=w1762, y=w1770) -> (x/y=w1768:dbl)
                      n809 = Reciprocal(x=w1768) -> (1/x=w1765:dbl)
                      n810 = Multiply(x=w1765, y=1000.0) -> (x*y=w1758:dbl)
                      n811 = Number To Fractional String(number=w1758, precision (6)=i16 2) -> (F-format string=w1754:string)  [unwired: 2 in]
                      n812 = Divide(x=w1765, y=9.81) -> (x/y=w1761:dbl)
                      n813 = In Range and Coerce(upper limit=14.5, x=w1758, lower limit=7.5) -> (In Range?=w1752:bool)  [unwired: 1 out]
                      n814 = Select(t="\n\nACCELEROMETER CALIBRATED CORRECTLY\n------------------------------------------------------------------------ \n", s=w1752, f="\n\nCALIBRATION FAILED\nSENSITIVITY OUT OF RANGE (7,5-14,5)\n------------------------------------------------------------------------ \n") -> (s? t:f=w1753:string)
                      n815 = Concatenate Strings("\nAMPLITUDE CALIBRATION:\n\nSENSIVITY: ", w1754, w1753, "\r") -> (w1751:string)
                    }
                  }
                  n816 = local read "Report"() -> (w1744:string)
                  n817 = Concatenate Strings(w1736, w1744) -> (w1743:string)
                  n818 = local write "Report"(w1743) -> ()
                  "Calibration parameter" <- w1741
                }
              }
              n819 = Wait Until Next ms Multiple(millisecond multiple=u32 200 ("milliseconds to wait")) -> ()  [unwired: 1 out]
              n820 = Not(x=w1035) -> (.not. x?=w1041:bool)
              n821 = Concatenate Strings(w1037, w1039) -> (w1038:string)
              "Numeric" <- w1036
            }
            n822 = while {
              tunnel: [w1012] -> w992
              tunnel: w993 -> [w1012]
              i -> [w1009]
              stop <- w1010 stop-if-true
              n823 = Wait (ms)(milliseconds to wait=u32 1000) -> ()  [unwired: 1 out]
              n824 = Greater?(x=w1009, y=2) -> (0:w1010:bool)
            }
            n825 = local read "calibration log"() -> (w999:path)
            n826 = Write to Text File(file (use dialog)=w999, text=w992) -> ()  [unwired: 2 in, 3 out]
            n827 = flat-sequence {
              tunnel: w998 -> [w1021]
              tunnel: w994 -> [w1020]
              tunnel: [w1021] -> w997
              tunnel: [w1020] -> w995
              frame #0 {
                # "Antes Accel. detected"
                n828 = local read "Accelerometer"() -> (w1018:i32)
                n829 = local read "Save calibration"() -> (w1017:bool)
                n830 = Add(x=w1018, y=7) -> (x+y=w1015:i32)
                n831 = Less Or Equal?(x=w1015, y=15) -> (x <= y?=w1016:bool)
                n832 = And(x=w1016, y=w1017) -> (x .and. y?=w1013:bool)
                n833 = case shown="True" w1013 {
                  tunnel: w1015 -> [_ w1022]
                  frame False {
                  }
                  frame True {
                    w1032 = "Parametros"  # Key 1
                    n834 = local read "configuration file path"() -> (w1024:path)
                    n835 = local read "Calibration parameter"() -> (w1023:dbl)
                    n836 = Number To Decimal String(number=w1022) -> (decimal integer string=w1033:string)  [unwired: 1 in]
                    n837 = Concatenate Strings(w1032, w1033) -> (w1026:string)
                    n838 = call <vilib>:"Open Config Data.vi"("create file if necessary (T)"=TRUE, "configuration file path"=w1024) -> ("error out"=w1027:errorcluster, "refnum"=w1028:T13)  [unwired: 1 in, 7 out]
                    n839 = call-poly <vilib>:"Write Key.vi"("section"="Adquisicion", "error in (no error)"=w1027, "value"=w1023, "key"=w1026, "refnum"=w1028) -> ("error out"=w1031:errorcluster, "refnum out"=w1030:T13)  [unwired: 3 in, 2 out]
                    n840 = call <vilib>:"Close Config Data.vi"("error in (no error)"=w1031, "refnum"=w1030) -> ()  [unwired: 8 in, 2 out]
                  }
                }
              }
            }
          }
          frame "UPS" {
            n841 = flat-sequence {
              tunnel: w1794 -> [w1806]
              tunnel: [w1806] -> w1793
              frame #0 {
                n842 = local read "Report"() -> (w1805:string)
                n843 = call "Reporting_datetime.vi"() -> ("String"=w1803:string)  [unwired: 11 in]
                n844 = Concatenate Strings(w1803, "\nSTATUS: UPS\n\n", w1805) -> (w1804:string)
                n845 = local write "Report"(w1804) -> ()
              }
            }
            n846 = node-c288() -> (w1801:T7)  [unwired: 4 in]
            n847 = timed-loop {
              timing: w1801 -> [_]
              timing-out: [_] -> w1800
              tunnel: w1799 -> [w1815]
              tunnel: w1793 -> [w1814]
              tunnel: [w1813] -> w1798
              tunnel: [w1812] -> w1797
              stop <- w1807 stop-if-true
              n848 = node-c288() -> ()  [unwired: 1 in, 1 out]
              n849 = xnode "Read/Write Control"("FPGA VI Reference In"=w1815, "error in"=w1814) -> ("FPGA VI Reference Out"=w1813:refnum<k20>, "error out"=w1812:errorcluster, "DC OK"=w1810:bool, "Chassis Temperature"=w1811:i16)
              n850 = call "ControlTemperatura.vi"("Chassis Temperature"=w1811) -> ("T fuera rango"=w1809:bool)  [unwired: 2 out]
              n851 = Not(x=w1809) -> (.not. x?=w1808:bool)
              n852 = And(x=w1810, y=w1808) -> (x .and. y?=w1807:bool)
              n853 = node-c288() -> ()  [unwired: 1 in, 1 out]
            }
            n854 = node-c288(w1800) -> ()  [unwired: 1 out]
          }
          frame "Diagnosis" {
            (unwired) "%Y/%m/%d %H:%M:%S" ("time format string (%c)")
            n855 = flat-sequence {
              tunnel: w1840 -> [w2049]
              tunnel: [w2049] -> w1839
              frame #0 {
                n856 = local read "Report"() -> (w2048:string)
                n857 = call "Reporting_datetime.vi"() -> ("String"=w2046:string)  [unwired: 11 in]
                n858 = Concatenate Strings(w2046, "\nSTATUS: AUTODIAGNOSIS\n\n", w2048) -> (w2047:string)
                n859 = local write "Report"(w2047) -> ()
              }
            }
            n860 = xnode "Invoke Method"("FPGA VI Reference In"=w1838, "error in"=w1839) -> ("FPGA VI Reference Out"=w1830:refnum<k20>, "error out"=w1831:errorcluster)  [unwired: 1 in]
            n861 = flat-sequence {
              tunnel: [w1863] -> w1837
              tunnel: [w1862] -> w1836
              tunnel: [w1853] -> w1835
              tunnel: [w1852] -> w1834
              tunnel: w1831 -> [w1864]
              tunnel: w1830 -> [w1851]
              tunnel: [w1844] -> w1826
              tunnel: [w1843] -> w1825
              tunnel: w1837 -> [w1888]
              tunnel: w1836 -> [w1889]
              tunnel: w1835 -> [w1886]
              tunnel: w1834 -> [w1885]
              tunnel: [w1887] -> w1833
              tunnel: [w1883] -> w1832
              tunnel: w1826 -> [w1878]
              tunnel: w1825 -> [w1877]
              tunnel: [w1874] -> w1824
              tunnel: w1833 -> [w1961]
              tunnel: w1832 -> [w1962]
              tunnel: w1824 -> [w1954]
              tunnel: [w1976] -> w1823
              tunnel: [w1975] -> w1822
              tunnel: [w2043] -> w1829
              tunnel: [w2044] -> w1820
              tunnel: w1823 -> [w2044]
              tunnel: w1822 -> [w2043]
              frame #0 {
                w1842 = sgl[] [] ("A1")
                n862 = local read "Frecuencia de muestreo y módulo CRIO"() -> (w1861:T3)
                n863 = local read "Escaneos de la FIFO por canal"() -> (w1858:u32)
                n864 = local read "Frecuencia de muestreo (Hz)"() -> (w1859:dbl)
                n865 = local read "Nº de acelerómetros"() -> (w1856:i32)
                n866 = Get Date/Time In Seconds() -> (seconds since 1Jan1904=→"Inicio diagnosis":timestamp)
                n867 = local read "Nº inductivos"() -> (w1857:i32)
                n868 = local read "Canal cero WS2"() -> (w1849:bool)
                n869 = local read "Canal cero WS1?"() -> (w1850:bool)
                n870 = local read "Count(mSec)"() -> (w1860:u32)
                n871 = xnode "Read/Write Control"("FPGA VI Reference In"=w1851, "error in"=w1864, "Fotocélula"=TRUE ("Adquirir")) -> ("FPGA VI Reference Out"=w1868:refnum<k20>, "error out"=w1867:errorcluster)
                n872 = Add(x=w1857, y=w1856) -> (x+y=w1855:i32)
                n873 = call "DMACalc.vi"("Number of Channels"=w1855, "Number of Samples"=w1858, "Rate (Hz)"=w1859) -> ("Block Size"=w1852:u32, "Time to Acquire Block (ms)"=w1853:i32, "Host Buffer Size"=w1854:u32)  [unwired: 6 in]
                n874 = xnode "Read/Write Control"("FPGA VI Reference In"=w1868, "error in"=w1867, "Data Rate"=w1861, "Digital?"=FALSE, "Count(mSec)"=w1860, "Canal cero WS1?"=w1850, "Canal cero WS2?"=w1849) -> ("FPGA VI Reference Out"=w1870:refnum<k20>, "error out"=w1869:errorcluster)
                n875 = xnode "Invoke Method"("FPGA VI Reference In"=w1870, "error in"=w1869, "Requested Depth"=w1854) -> ("FPGA VI Reference Out"=w1872:refnum<k20>, "error out"=w1871:errorcluster)  [unwired: 1 out]
                n876 = Open/Create/Replace File(file path (use dialog)=path "c:/diagnosis.bin" ("file (use dialog)"), operation (0:open)=T5."replace or create", access (0:read/write)=enum16{"read/write", "read-only", "write-only"}."read/write", disable buffering (F)=TRUE) -> (refnum out=w1844:refnum<file>, error out=w1843:errorcluster)  [unwired: 1 in, 2 out]
                n877 = xnode "Invoke Method"("FPGA VI Reference In"=w1872, "error in"=w1871) -> ("FPGA VI Reference Out"=w1863:refnum<k20>, "error out"=w1862:errorcluster)
                n878 = local write "A1"(w1842) -> ()
                n879 = local write "A2"(w1842) -> ()
                n880 = local write "A3"(w1842) -> ()
                n881 = local write "A4"(w1842) -> ()
                n882 = local write "A5"(w1842) -> ()
                n883 = local write "A6"(w1842) -> ()
                n884 = local write "A7"(w1842) -> ()
                n885 = local write "A8"(w1842) -> ()
                n886 = local write "I1"(w1842) -> ()
                n887 = local write "I2"(w1842) -> ()
              }
              frame #1 {
                n888 = while "Data Acquisition" {
                  tunnel: w1888 -> [w1917]
                  shift-right: [w1921] -> _
                  shift-left: u32 0 ("t") -> [w1896]
                  tunnel: w1886 -> [w1922]
                  tunnel: w1885 -> [w1920]
                  shift-right: [w1923] -> w1883
                  shift-left: w1889 -> [w1916]
                  tunnel: [w1918] -> w1887
                  tunnel: w1878 -> [w1894]
                  shift-right: [w1891] -> w1876
                  shift-left: w1877 -> [w1893]
                  tunnel: [w1892] -> w1875
                  stop <- w1919 stop-if-true
                  # "Detector de presencia"
                  # "Mide el tiempo de paso del tren y con ello se puede calcular\nla velocidad la unidad"
                  n889 = xnode "Invoke Method"("FPGA VI Reference In"=w1917, "error in"=w1916, "Number of Elements"=w1896, "Timeout (ms)"=0) -> ("FPGA VI Reference Out"=w1909:refnum<k20>, "error out"=w1908:errorcluster, "Data"=w1915:fxp<+/-,24,4>[], "Elements Remaining"=w1897:u32)
                  n890 = case "Data Ready" shown="Default" w1896 {
                    tunnel: w1922 -> [w1928 _]
                    tunnel: [w1926 u32 0 ("t")] -> w1921
                    tunnel: w1920 -> [w1929 _]
                    tunnel: w1897 -> [w1927 _]
                    tunnel: w1915 -> [_ w1943]
                    tunnel: w1893 -> [w1925 w1940]
                    tunnel: [w1925 w1938] -> w1891
                    tunnel: w1894 -> [w1924 w1937]
                    tunnel: [w1924 w1936] -> w1892
                    frame 0 {
                      n891 = Greater Or Equal?(x=w1927, y=w1929) -> (x >= y?=w1930:bool)
                      n892 = case shown="False" w1930 {
                        tunnel: [u32 0 ("Block Size") w1934] -> w1926
                        tunnel: [w1933 0 ("t")] -> w1931
                        tunnel: w1928 -> [w1933 _]
                        tunnel: w1929 -> [_ w1934]
                        frame False {
                        }
                        frame True {
                        }
                      }
                      n893 = call "WaitMinTimeBetweenCall.vi"("Minimum ms between calls"=w1931) -> ()  [unwired: 2 in]
                    }
                    frame Default {
                      n894 = To Single Precision Float(number=w1943) -> (single precision float=w1939:sgl[])
                      n895 = Write to Binary File(file (use dialog)=w1937, data=w1939, error in=w1940, 5:FALSE ("prepend array or string size? (T)"), 9:T6."little-endian" ("byte order (0:big-endian, network order)")) -> (refnum out=w1936:refnum<file>, error out=w1938:errorcluster)  [unwired: 2 out]
                    }
                  }
                  n896 = xnode ("CheckLate")("FPGA VI Reference In"=w1909, "error in"=w1908) -> ("FPGA VI Reference Out"=w1904:refnum<k20>, "error out"=w1913:errorcluster, "Buffer Underflow"=w1899:bool, "Buffer Overflow"=w1900:bool)
                  n897 = local read "Inicio diagnosis"() -> (w1901:timestamp)
                  n898 = Get Date/Time In Seconds() -> (seconds since 1Jan1904=w1902:timestamp)
                  n899 = To Double Precision Float(number=w1901) -> (double precision float=w1907:dbl)
                  n900 = To Double Precision Float(number=w1902) -> (double precision float=w1906:dbl)
                  n901 = local write "Buffer Overflow"(w1900) -> ()
                  n902 = Subtract(x=w1906, y=w1907) -> (x-y=w1910:dbl)
                  n903 = local write "Buffer Underflow"(w1899) -> ()
                  n904 = Greater?(x=w1910, y=1.0 ("Tiempo de adquisición")) -> (0:w1905:bool)
                  n905 = call "ErrorOverFlow.vi"("Buffer Overflow"=w1900) -> ("error out"=w1911:errorcluster)
                  n906 = call "ErrorUnderFlow.vi"("Buffer Overflow"=w1899) -> ("error out"=w1912:errorcluster)
                  n907 = Unbundle By Name(w1891) -> ("status"=w1890:bool)
                  n908 = Merge Errors(w1913, w1912, w1911) -> (w1895:errorcluster)
                  n909 = Unbundle By Name(w1895) -> ("status"=w1914:bool)
                  n910 = Compound Arithmetic op=OR(w1914, w1905, w1890) -> (w1919:bool)
                  n911 = case "Flush" shown="True" w1919 {
                    tunnel: w1904 -> [w1945 w1950]
                    tunnel: w1895 -> [w1946 w1949]
                    tunnel: [w1946 w1948] -> w1923
                    tunnel: [w1945 w1947] -> w1918
                    frame False {
                    }
                    frame True {
                      n912 = xnode "Invoke Method"("FPGA VI Reference In"=w1950, "error in"=w1949) -> ("FPGA VI Reference Out"=w1947:refnum<k20>, "error out"=w1948:errorcluster)
                    }
                  }
                }
                n913 = local read "Report"() -> (w1882:string)
                n914 = call "Reporting_error.vi"("error out 2"=w1883, "Concept"="FPGA ") -> ("Reporting"=w1884:string)  [unwired: 1 in]
                n915 = Close File(refnum=w1875, error in=w1876) -> (path=w1874:path)  [unwired: 1 out]
                n916 = Concatenate Strings(w1884, w1882) -> (w1879:string)
                n917 = local write "Report"(w1879) -> ()
              }
              frame #2 {
                n918 = xnode "Read/Write Control"("FPGA VI Reference In"=w1961, "error in"=w1962) -> ("FPGA VI Reference Out"=w1959:refnum<k20>, "error out"=w1960:errorcluster, "Direccion 0?"=w1958:bool)
                n919 = Read from Binary File(5:sgl 1.25, 9:T6."little-endian" ("byte order (0:big-endian, network order)"), 10:-1 ("count (1)"), 11:w1954) -> (0:w1952:errorcluster, 2:w1953:sgl[], 3:w1951:refnum<file>)  [unwired: 1 in, 2 out]
                "Diagnostic data" <- w1953
                n920 = local write "Direccion 0?"(w1958) -> ()
                n921 = Close File(refnum=w1951, error in=w1952) -> ()  [unwired: 2 out]
                n922 = Decimate 1D Array(w1953) -> (w1967:sgl[], w1964:sgl[], w1965:sgl[], w1966:sgl[], w1968:sgl[], w1969:sgl[], w1970:sgl[], w1971:sgl[], w1972:sgl[], w1973:sgl[])
                n923 = Build Array(w1967, w1964, w1965, w1966, w1968, w1969, w1970, w1971, w1972, w1973) -> (w1963:sgl[][])
                n924 = xnode "Read/Write Control"("FPGA VI Reference In"=w1959, "error in"=w1960, "Stop"=TRUE) -> ("FPGA VI Reference Out"=w1977:refnum<k20>, "error out"=w1978:errorcluster)
                n925 = for {
                  tunnel: w1963 -> [w1979] mode=indexing
                  i -> [w1980]
                  n926 = case shown="9" w1980 {
                    tunnel: w1979 -> [w1981 w1982 w1983 w1984 w1985 w1986 w1987 w1988 w1989 w1990 _]
                    frame 0 {
                      "A1" <- w1981
                    }
                    frame 1 {
                      "A2" <- w1982
                    }
                    frame 2 {
                      "A3" <- w1983
                    }
                    frame 3 {
                      "A4" <- w1984
                    }
                    frame 4 {
                      "A5" <- w1985
                    }
                    frame 5 {
                      "A6" <- w1986
                    }
                    frame 6 {
                      "A7" <- w1987
                    }
                    frame 7 {
                      "A8" <- w1988
                    }
                    frame 8 {
                      "I1" <- w1989
                    }
                    frame 9 {
                      "I2" <- w1990
                    }
                    frame 10, Default {
                    }
                  }
                }
                n927 = xnode "Invoke Method"("FPGA VI Reference In"=w1977, "error in"=w1978) -> ("FPGA VI Reference Out"=w1976:refnum<k20>, "error out"=w1975:errorcluster)
              }
              frame #3 {
                n928 = local read "Puerto RFID"() -> (w2037:u16)
                n929 = local read "configuration file path"() -> (w2030:path)
                n930 = local read "IP RFID"() -> (w2038:string)
                n931 = local read "RFID_status"() -> (w2040:path)
                n932 = call "Read_diagnosis_data.vi"("configuration file path"=w2030) -> ("acelerometros"=w2021:dbl, "WD"=w2034:dbl)  [unwired: 9 in]
                n933 = call "conexion_internet.vi"() -> ("Internet status"=w2004:string, "Internet connection"=→"Internet connection":bool)  [unwired: 10 in]
                n934 = call "RFID_connection.vi"("Puerto RFID"=w2037, "IP RFID"=w2038) -> ("RFID_connection_text"=w2003:string, "RFID connection"=→"RFID connection":bool)  [unwired: 8 in]
                n935 = call "show_tag_status.vi"("file path (dialog if empty)"=w2040) -> ("Output"=→"Last Train passes - RFIDs":T1, "train_passes_text"=w2002:string)  [unwired: 9 in]
                n936 = local read "Direccion 0?"() -> (w2033:bool)
                n937 = local read "I1"() -> (w2032:sgl[])
                n938 = local read "I2"() -> (w2031:sgl[])
                n939 = local read "A1"() -> (w2020:sgl[])
                n940 = local read "A2"() -> (w2019:sgl[])
                n941 = local read "A3"() -> (w2013:sgl[])
                n942 = local read "A4"() -> (w2014:sgl[])
                n943 = local read "A5"() -> (w2015:sgl[])
                n944 = local read "A6"() -> (w2016:sgl[])
                n945 = local read "A7"() -> (w2017:sgl[])
                n946 = local read "A8"() -> (w2018:sgl[])
                n947 = call "Wheel_detector_status.vi"("WD_offset"=w2034, "I2"=w2031, "I1"=w2032, "Direccion 0?"=w2033) -> ("WD_status"=w2001:string, "I2"=→"Wheel detector 2":bool, "I1"=→"Wheel Detector 1":bool)  [unwired: 5 in]
                n948 = call "Accelerometer_status.vi"("Number"=1, "Acc_offset"=w2021, "Accelerometer"=w2020) -> ("Accelerometer_status"=w2000:string, "Accelerometer"=→"Accelerometer 1":bool)  [unwired: 7 in]
                n949 = call "Accelerometer_status.vi"("Number"=2, "Acc_offset"=w2021, "Accelerometer"=w2019) -> ("Accelerometer_status"=w1999:string, "Accelerometer"=→"Accelerometer 2":bool)  [unwired: 7 in]
                n950 = call "Accelerometer_status.vi"("Number"=3, "Acc_offset"=w2021, "Accelerometer"=w2013) -> ("Accelerometer_status"=w1998:string, "Accelerometer"=→"Accelerometer 3":bool)  [unwired: 7 in]
                n951 = call "Accelerometer_status.vi"("Number"=4, "Acc_offset"=w2021, "Accelerometer"=w2014) -> ("Accelerometer_status"=w1997:string, "Accelerometer"=→"Accelerometer 4":bool)  [unwired: 7 in]
                n952 = call "Accelerometer_status.vi"("Number"=5, "Acc_offset"=w2021, "Accelerometer"=w2015) -> ("Accelerometer_status"=w1996:string, "Accelerometer"=→"Accelerometer 5":bool)  [unwired: 7 in]
                n953 = call "Accelerometer_status.vi"("Number"=6, "Acc_offset"=w2021, "Accelerometer"=w2016) -> ("Accelerometer_status"=w1995:string, "Accelerometer"=→"Accelerometer 6":bool)  [unwired: 7 in]
                n954 = call "Accelerometer_status.vi"("Number"=7, "Acc_offset"=w2021, "Accelerometer"=w2017) -> ("Accelerometer_status"=w1994:string, "Accelerometer"=→"Accelerometer 7":bool)  [unwired: 7 in]
                n955 = call "Accelerometer_status.vi"("Number"=8, "Acc_offset"=w2021, "Accelerometer"=w2018) -> ("Accelerometer_status"=w1993:string, "Accelerometer"=→"Accelerometer 8":bool)  [unwired: 7 in]
                n956 = local read "Report"() -> (w1992:string)
                n957 = Concatenate Strings(w2004, w2003, w2002, w2001, w2000, w1999, w1998, w1997, w1996, w1995, w1994, w1993, w1992) -> (w1991:string)
                n958 = property on="Report" class="Str"("Value"=w1991) -> ()  [unwired: 2 in, 2 out]
              }
            }
            n959 = Get Date/Time In Seconds() -> (seconds since 1Jan1904=w1828:timestamp)
            n960 = Format Date/Time String(seconds (now)=w1828) -> (date/time string=→"Last time checked":string)  [unwired: 2 in]
          }
        }
        "error manipulacion archivos" <- w111
        "t" <- w107
        n961 = local read "Parar la aplicación"() -> (w109:bool)
      }
      n962 = case shown="True" w82 {
        frame False {
        }
        frame True {
          w90 = T14 {"IP"="169.254.1.1", "Port"=5084, "ReaderConfigFile"=path "", "ROspecConfigFile"=path ""}  # RFID Configuration
          w94 = path "" ("ReaderConfigFile")
          # "Loop RFID reader"
          n963 = local read "Puerto RFID"() -> (w92:u16)
          n964 = local read "IP RFID"() -> (w93:string)
          n965 = Bundle By Name(cluster=w90, "IP"=w93, "Port"=w92, "ReaderConfigFile"=w94, "ROspecConfigFile"=w94) -> (w91:T14)
          n966 = while {
            tunnel: w91 -> [w96]
            stop <- w97 stop-if-true
            n967 = local read "Parar la aplicación"() -> (w97:bool)
            n968 = call "IF2_Reader.vi"("Stop"=w97, "RFID Configuration"=w96) -> ("error out"=w98:errorcluster, "connection ID"=→"connection ID":refnum<k5>)  [unwired: 8 in]
            n969 = case shown="Error" w98 {
              tunnel: w98 -> [_ w100]
              tunnel: [TRUE ("RFIDStatus") FALSE ("RFIDStatus")] -> _
              frame No Error {
              }
              frame Error {
                n970 = call "Reporting_error.vi"("error out 2"=w100, "Concept"="Passive RFID") -> ("Reporting"=w102:string)  [unwired: 1 in]
                n971 = local read "Report"() -> (w103:string)
                n972 = Concatenate Strings(w102, w103) -> (w101:string)
                n973 = local write "Report"(w101) -> ()
              }
            }
          }
        }
      }
      n974 = xnode "Close FPGA VI Reference"("FPGA VI Reference In"=w85, "error in"=w84) -> ("error out"=→"error FPGA":errorcluster)
    }
    frame #3 {
      n975 = call "LH6HD.vi"("Action"=enum16{"Init", "Start", "Read", "Stop", "Exit"}."Stop") -> ("error out"=→"RFID_LR6_Error":errorcluster)  [unwired: 9 in, 1 out]
    }
  }
